vi "Camera Main.vi"() -> ()   [LabVIEW 2013]
uses:
  Controls/Controls Tab.ctl
  <vilib>/Utility/miscctls.llb/LVRectTypeDef.ctl
  GUI_Template/GUI_master/tcp_new_data_event.ctl
  GUI_Template/GUI_master/tcp new data cluster.ctl
  color tables/image color table presets.ctl
  Controls/IMAQ control.ctl
  <vilib>/vision/Image Controls.llb/IMAQ Image.ctl
  Controls/IMG Features.ctl
  Controls/TCP Cluster.ctl
  <vilib>/vision/NI_Vision_Development_Module.lvlib
panel:
  out "fast ID (h)":refnum<k16>
  out "slow ID (h)":refnum<k16>
  in  "Color table":T1=enum."BWR enhance low"
  in  "Maximize!!":bool
  out "error message":string
  out "Device Name (h)":string="FakeCam1"
  in  "Hide controls":bool
  out "image::1":T2(plugin-control) caption="HPD_CCD"
  in  "File Path":path
  out "error IO 2":errorcluster
  out "tcp data event":T3
  in  "Tab Control":T4
  in  "size 2":cluster{"xhair size":dbl, "xhair size 2":dbl}={"xhair size"=20.0, "xhair size 2"=20.0} {"xhair size 2" min=0.0 max=0.0; "xhair size" min=0.0 max=0.0}
  in  "Target.X":dbl caption="TargetX"
  in  "Target.Y":dbl caption="TargetY"
  in  "draw Xhair":bool
  in  "Scale":bool
  in  "Autoscale":bool
  in  "String":string="M1Cam"
  in  "GUIdevice 1":string="HPD_CCD"
  in  "stop":bool
  in  "scale factor":dbl=2.0 caption="Scale factor"
  in  "Trigger":bool
  in  "Save":bool
  in  "Gain":dbl
  in  "exposure":dbl=0.52 caption="Exposure"
  in  "Triggerdelay":dbl
  in  "Fit Control":bool
  in  "Shotnumber":i32=354
  out "Max Counts":dbl(slide) scale=0.0..256.0
  in  "Size & Tolerance":T5={"X Size"=5, "Y Size"=5, "% Tolerance"=100}
  in  "LowPass":bool
  in  "Sat Level":sgl=255.0
  out "Mean Value":sgl format="%.2f"
  in  "Beep If Sat.":bool
  in  "MaxGUIPixel":dbl
  in  "ROI.Width":dbl
  in  "ROI.Height":dbl
  in  "ROI.OffsetX":dbl
  in  "ROI.OffsetY":dbl
  out "Centroid":cluster{"X Centroid":sgl, "Y Centroid":sgl} {"Y Centroid" format="%.2f"; "X Centroid" format="%.2f"}
  out "Y Resolution":i32
  out "X Resolution":i32
  out "GUIBinning":dbl
  out "Mean Value Graph":sgl(graph)
  out "histogram":T6(graph)
  out "lineout":cluster{"x0":sgl, "dx":sgl, "Pixels Line":sgl[]}(graph)
  out "MaxCounts":dbl
  in  "SpatialCalibration":dbl
  in  "FWHMx":dbl
  in  "FWHMy":dbl
  out "FWHMx (um)":dbl
  out "FWHMy (um)":dbl
  in  "Analysis":bool
  out "MeanCounts":dbl
  in  "localsavingpath":path
  in  "time to wait (TCP)":i32=10
  in  "send":bool
  in  "reset":bool
  in  "Timeout ms (slow resp)":i32=500
  out "port or service name":u16=65400
  out "local Port":u16=65401
  out "connections (hidden)":variant[](array[variant])=[variant(refnum<k16> refnum), variant(refnum<k16> refnum)]
  out "Data connection ok":bool
  out "Image connection":bool
  out "error (h)":bool
  out "centroidy 2":dbl
  out "centroidy":dbl
  out "Remote Host":string="192.168.10.157"
  out "Top":i16
  out "Left":i16
  out "Content Area Rect":T7
  out "Image (IMAQ)":T2(plugin-control)
  # "Unused controls Do not Delete"
  # "Crosshair"
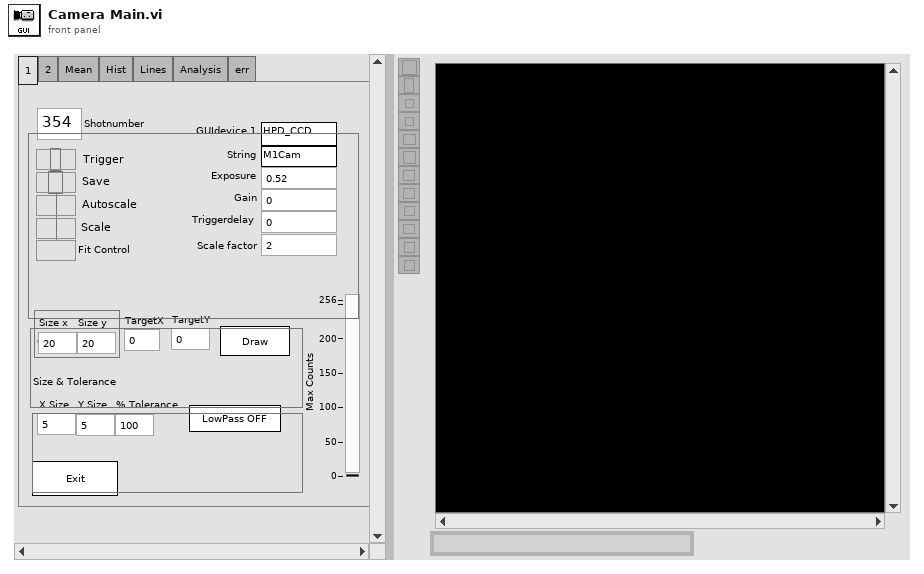
[diagram p1: front panel]
types:
  T1 = typedef "image color table presets.ctl" = enum16{"enhance low", "blue yellow red", "BYR enhance low", "white blue yellow", "BWR enhance low", "make a new one"}
  T2 = typedef "IMAQ Image.ctl" = refnum<image>
  T3 = typedef "tcp_new_data_event.ctl" = refnum<user-event>
  T4 = typedef "Controls Tab.ctl" = enum32{"1", "2", "Mean", "Hist", "Lines", "Analysis", "err"}
  T5 = cluster{"X Size":i32, "Y Size":i32, "% Tolerance":i32}
  T6 = cluster{"Starting Value":sgl, "Incremental Value":sgl, "Histogram":u32[]}
  T7 = typedef "LVRectTypeDef.ctl" = cluster{"Left":i16, "Top":i16, "Right":i16, "Bottom":i16}
  T8 = typedef "EventTypDef.ctl" = refnum<user-event>
  T9 = enum32{"Invalid", "Standard", "Closed", "Hidden", "Minimized", "Maximized"}
  T10 = enum32{"invalid app kind", "Development System", "Run Time System", "Student Edition", "Embedded LabVIEW", "Evaluation", "Custom"}
  T11 = cluster{"Left":i32, "Top":i32, "Right":i32, "Bottom":i32}
  T12 = typedef "IMAQ control.ctl" = cluster{"Image Out":T2, "valid image":bool, "X resolution":i32, "Y resolution":i32, "Image Area":cluster{"Width":u32, "Height":u32}, "zoom to fit":bool, "Image Center":cluster{"X":u32, "Y":u32}, "Max count":dbl}
  T13 = typedef "IMG Features.ctl" = cluster{"Color table":T1, "Button Label":string}
  T14 = typedef "TCP Cluster.ctl" = cluster{"Port":u16, "Remote Host":string, "All Devices":string[], "New Device":bool}
  T15 = cluster{"Core":cluster{"Current VI Reference":refnum<vi>, "Close Panel on Exit?":bool}, "tcp connections":refnum<k5>[], "subscribe messages":string[], "Image Data":T12, "images":T2[], "IMG Features":T13, "TCP Cluster":T14}
  T16 = typedef "Image Type" = u32
  T17 = cluster{"Current VI Reference":refnum<vi>, "Close Panel on Exit?":bool}
  T18 = cluster{"Global Rectangle":i32[], "Contours":cluster{"Contour Type":u32, "ROI Type":u32, "Points":i32[]}[]}
  T19 = typedef "IMAQ Line" = cluster{"Start X":i32, "Start Y":i32, "End X":i32, "End Y":i32}
  T20 = typedef "tcp new data cluster.ctl" = cluster{"EventEnum":enum16{"new data", "connection status update"}, "Device name":string}
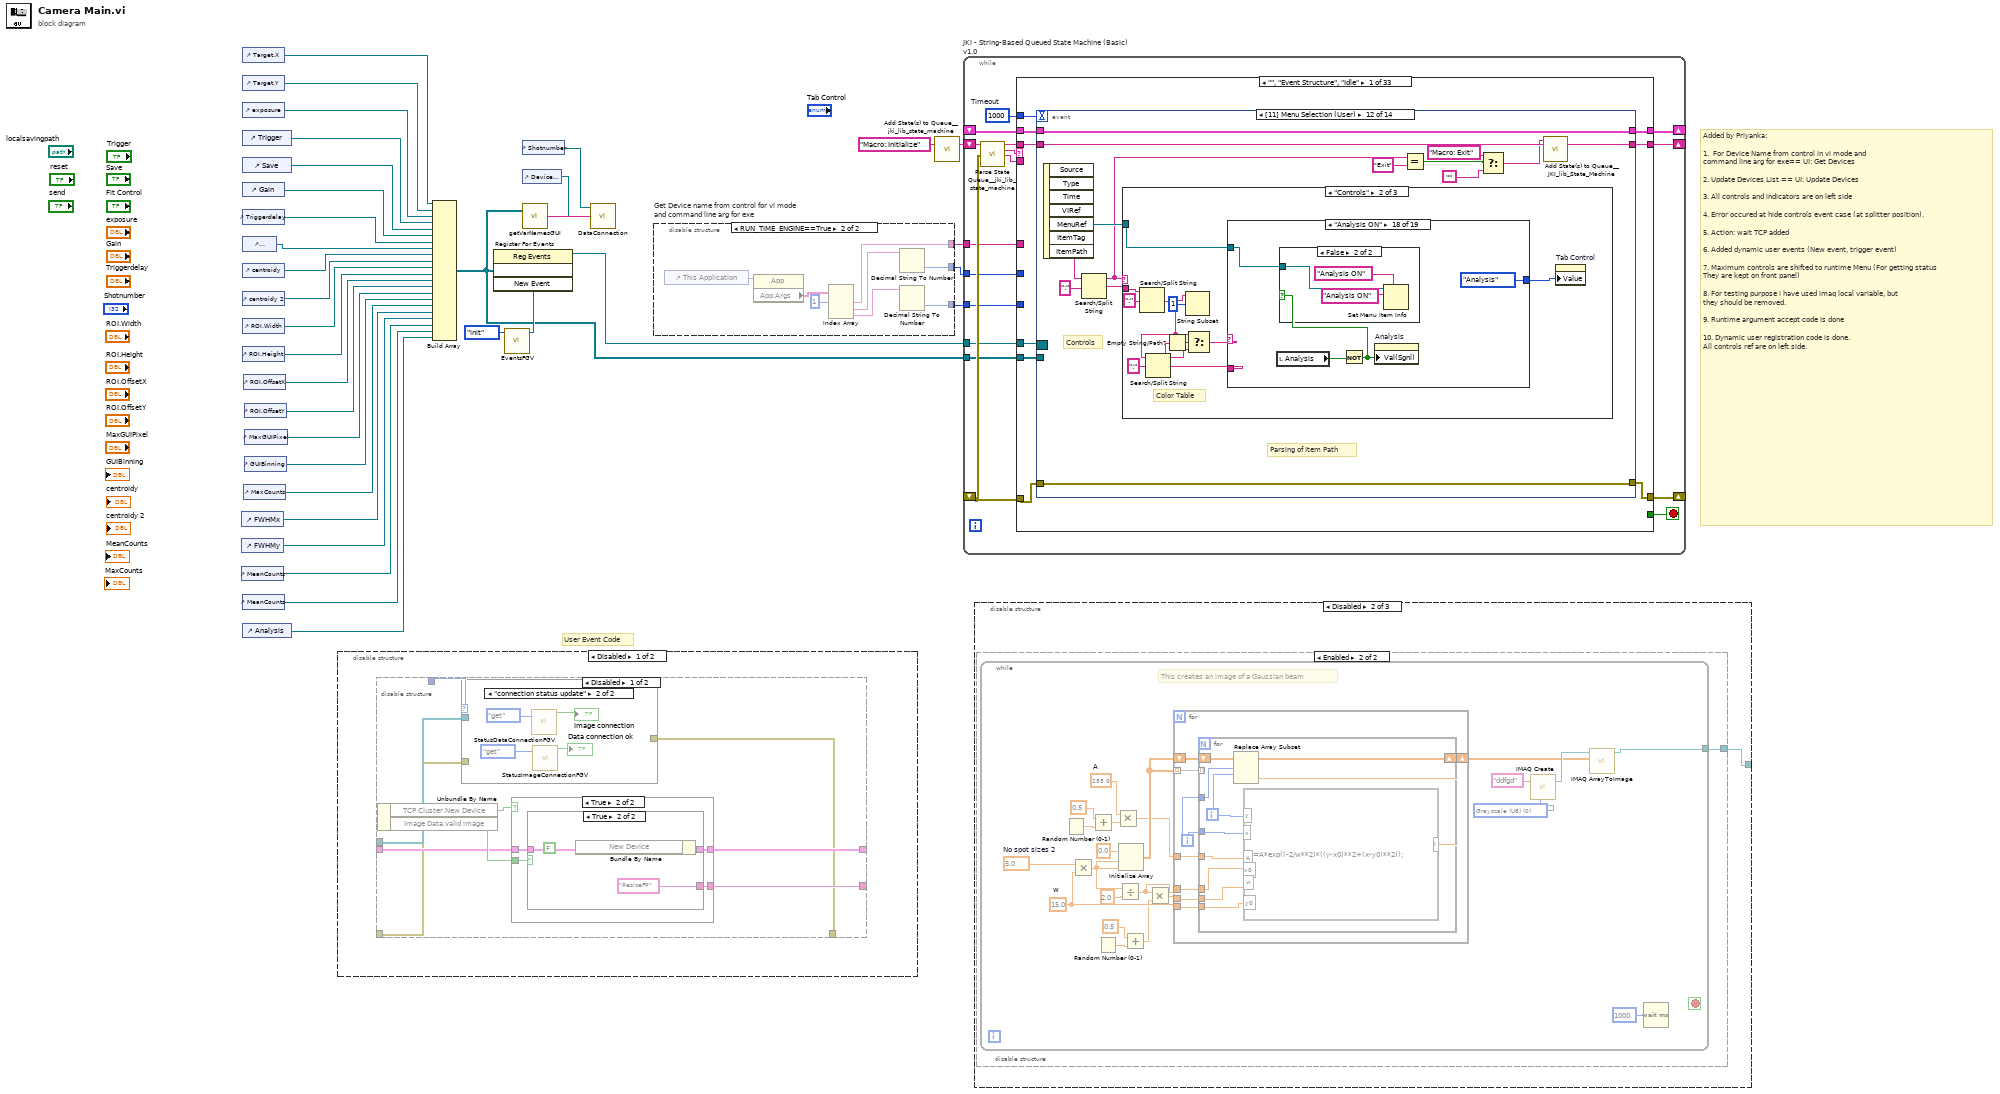
[diagram p0: block diagram]
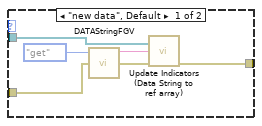
[diagram p4: hidden frame]
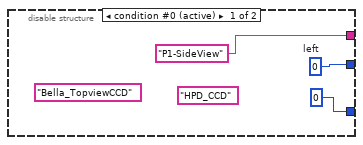
[diagram p7: hidden frame]
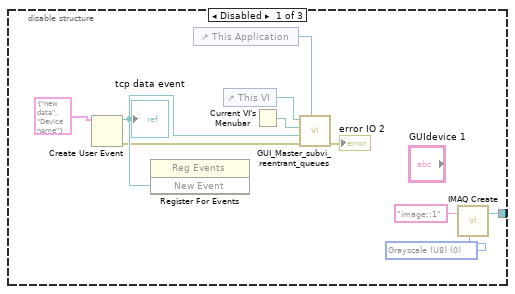
[diagram p8: hidden frame]
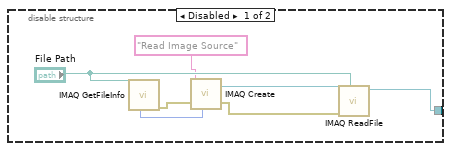
[diagram p9: hidden frame]
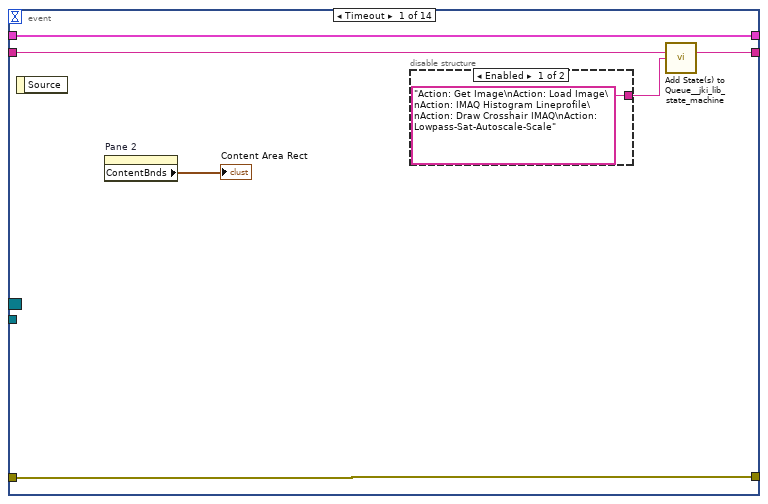
[diagram p11: hidden frame]
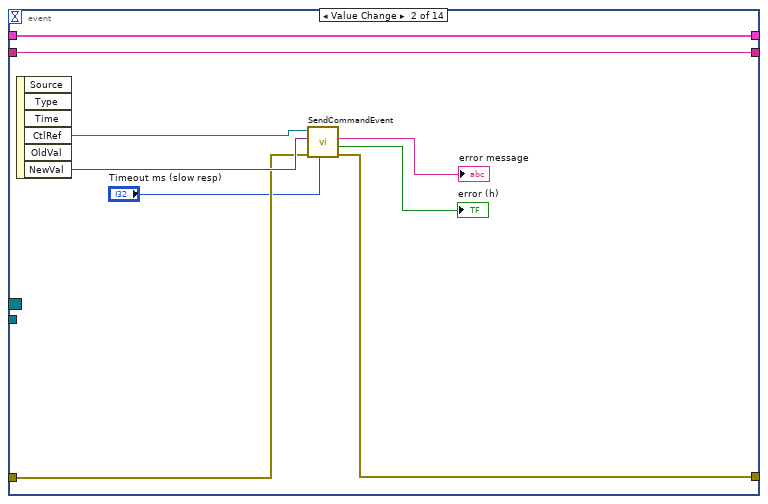
[diagram p13: hidden frame]
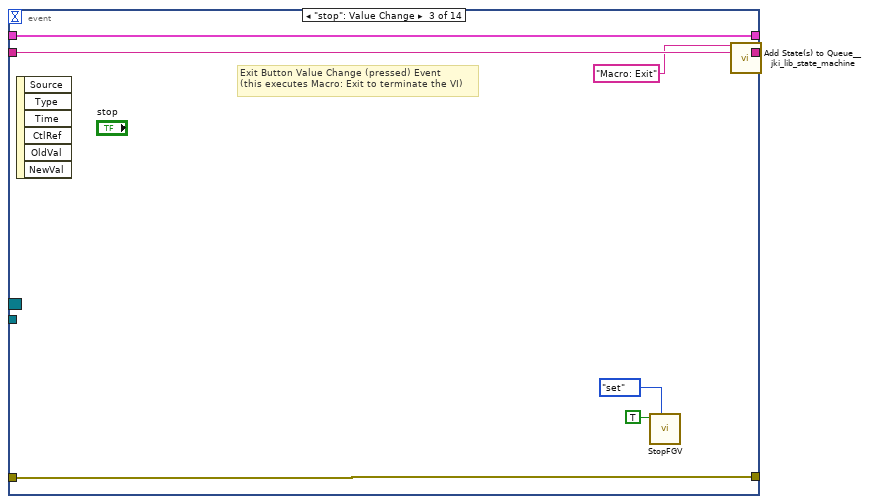
[diagram p14: hidden frame]
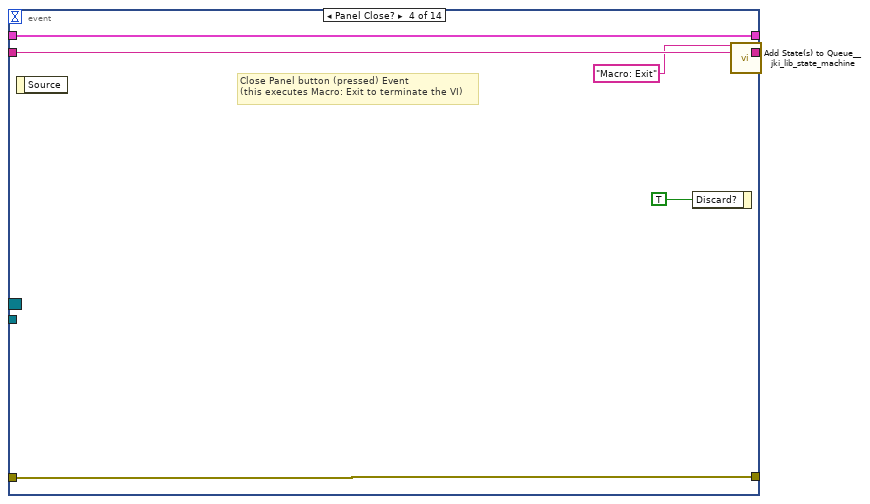
[diagram p15: hidden frame]
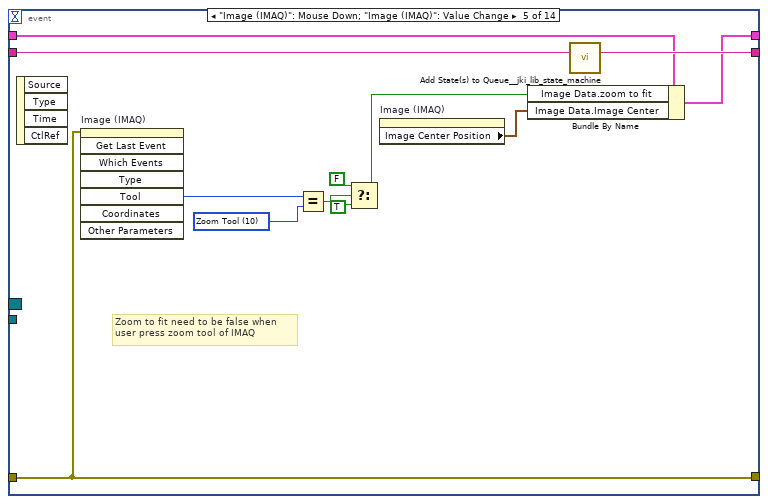
[diagram p16: hidden frame]
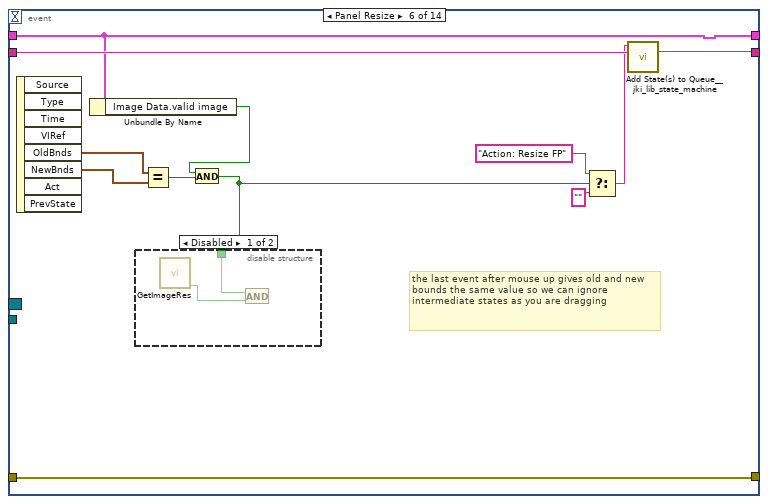
[diagram p17: hidden frame]
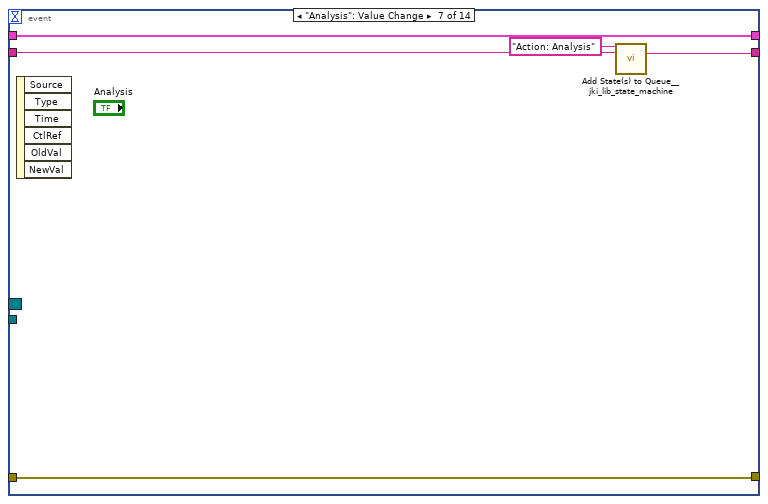
[diagram p19: hidden frame]
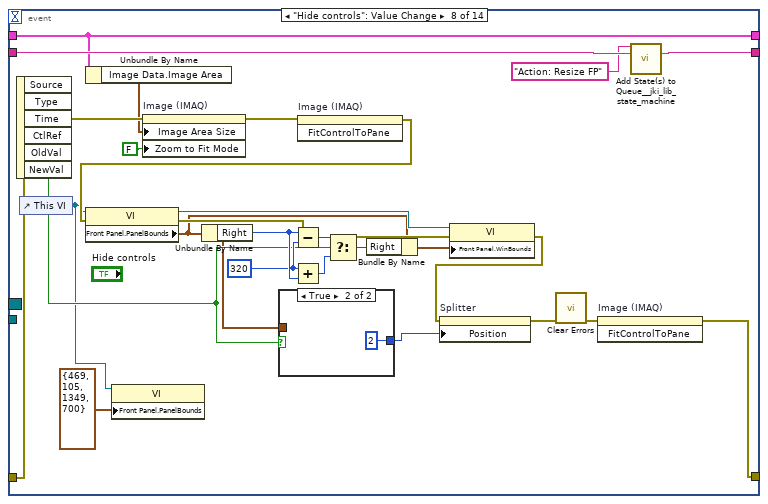
[diagram p20: hidden frame]
diagram:
  # "User Event Code"
  # "Added by Priyanka:\n\n1.  For Device Name from control in vi mode and \ncommand line arg for exe== UI: Get Devices\n\n2. Update Devices List == UI: Update Devices\n\n3. All controls and indicators are on left side\n\n4. Error occured at hide controls event case (at splitter position).\n\n5. Action: wait TCP added\n\n6. Added dynamic user events (New event, trigger event)\n\n7. Maximum controls are shifted to runtime Menu (For getting status\nThey are kept on front panel)\n\n8. For testing purpose i have used imaq local variable, but \nthey should be removed.\n\n9. Runtime argument accept code is done\n\n10. Dynamic user registration code is done. \nAll controls ref are on left side."
  n1 = control-ref of="FWHMx"() -> (w9:refnum<vi>)
  n2 = control-ref of="FWHMy"() -> (w8:refnum<vi>)
  n3 = control-ref of="MeanCounts"() -> (w7:refnum<vi>)
  n4 = control-ref of="Target.X"() -> (w26:refnum<vi>)
  n5 = control-ref of="Target.Y"() -> (w25:refnum<vi>)
  n6 = control-ref of="exposure"() -> (w24:refnum<vi>)
  n7 = control-ref of="Trigger"() -> (w23:refnum<vi>)
  n8 = control-ref of="Save"() -> (w22:refnum<vi>)
  n9 = control-ref of="Gain"() -> (w21:refnum<vi>)
  n10 = control-ref of="Triggerdelay"() -> (w20:refnum<vi>)
  n11 = control-ref of="localsavingpath"() -> (w15:refnum<vi>)
  n12 = control-ref of="centroidy"() -> (w19:refnum<vi>)
  n13 = control-ref of="centroidy 2"() -> (w18:refnum<vi>)
  n14 = control-ref of="ROI.Width"() -> (w17:refnum<vi>)
  n15 = control-ref of="ROI.Height"() -> (w16:refnum<vi>)
  n16 = control-ref of="MeanCounts"() -> (w6:refnum<vi>)
  n17 = control-ref of="Analysis"() -> (w5:refnum<vi>)
  n18 = control-ref of="ROI.OffsetX"() -> (w14:refnum<vi>)
  n19 = control-ref of="MaxCounts"() -> (w10:refnum<vi>)
  n20 = control-ref of="ROI.OffsetY"() -> (w13:refnum<vi>)
  n21 = control-ref of="GUIBinning"() -> (w11:refnum<vi>)
  n22 = control-ref of="MaxGUIPixel"() -> (w12:refnum<vi>)
  n23 = disable-structure shown="Disabled" {
    frame Disabled {
      n24 = disable-structure shown="Disabled" {
        disable-tunnel: _ -> [w43 _]
        disable-tunnel: _ -> [w42 _]
        disable-tunnel: [w39 _] -> _
        disable-tunnel: _ -> [w38 _]
        disable-tunnel: [w37 _] -> _
        disable-tunnel: [w36 _] -> _
        disable-tunnel: _ -> [w35 _]
        frame Disabled {
          n25 = Unbundle By Name() -> ("TCP Cluster.New Device"=w40:bool, "Image Data.valid image"=w41:bool)  [unwired: 1 in]
          n26 = case shown="\"connection status update\"" w42 {
            tunnel: w43 -> [w57 _]
            tunnel: [w55 _] -> w36
            tunnel: w35 -> [w54 _]
            frame "new data", Default {
              n27 = call "DATAStringFGV.vi"("Command"=enum16{"get", "set", "init"}."get") -> ("Data String out"=w56:string)  [unwired: 9 in, 1 out]
              n28 = call "Update Indicators (Data String to ref array).vi"("Array"=w57, "Data String"=w56, "error in (no error)"=w54) -> ("error out"=w55:errorcluster)  [unwired: 11 in, 1 out]
            }
            frame "connection status update" {
              n29 = call "StatusDataConnectionFGV.vi"("Command"=enum16{"get", "set", "init"}."get") -> ("Data Connection out"=→"Image connection":bool)  [unwired: 10 in]
              n30 = call "StatusImageConnectionFGV.vi"("Command"=enum16{"get", "set", "init"}."get") -> ("Image Connection out"=→"Data connection ok":bool)  [unwired: 10 in]
            }
          }
          n31 = case shown="True" w40 {
            tunnel: [_ w48] -> w39
            tunnel: w41 -> [_ w47]
            tunnel: w38 -> [w44 w46]
            tunnel: [w44 w45] -> w37
            frame False {
            }
            frame True {
              n32 = case shown="True" w47 {
                tunnel: [_ "ResizeFP" ("State(s) in (\"\")")] -> w48
                tunnel: w46 -> [w49 w52]
                tunnel: [w49 w51] -> w45
                frame False {
                }
                frame True {
                  n33 = Bundle By Name(cluster=w52, "New Device"=FALSE ("new device")) -> (w51:cluster{})
                }
              }
            }
          }
        }
        frame Enabled {
        }
      }
    }
    frame Enabled {
    }
  }
  n34 = Build Array(w26, w25, w24, w23, w22, w21, w20, w15, w19, w18, w17, w16, w14, w13, w12, w11, w10, w9, w8, w7, w6, w5) -> (w3:refnum<vi>[])
  n35 = call "EventsFGV.vi"("Command"=enum16{"get", "init"}."init") -> ("New Event"=w27:T8)  [unwired: 9 in, 1 out]
  n36 = register-events(w3, w27) -> (reference out=w4:refnum<event-registration>)  [unwired: 2 in, 1 out]
  n37 = control-ref of="Shotnumber"() -> (w2:refnum<vi>)
  n38 = control-ref of="Device Name (h)"() -> (w1:refnum<vi>)
  n39 = call "getVarNamesGUI.vi"("Array"=w3) -> ("String"=w29:string)  [unwired: 1 in]
  n40 = call "DataConnection.vi"("Subscriber list"=w29, "Device Name (h)"=w1, "shotnumber"=w2) -> ()
  n41 = disable-structure "Get Device name from control for vi mode\nand command line arg for exe" shown="RUN_TIME_ENGINE==True" {
    disable-tunnel: ["P1-SideView" ("Device Name for vi mode") w70] -> w32
    disable-tunnel: [w64 w67] -> w30
    disable-tunnel: [i16 0 ("left") w66] -> w31
    frame condition #0 (active) {
      (unwired) "Bella_TopviewCCD" ("Device Name for vi mode")
      (unwired) "HPD_CCD" ("Device Name for vi mode")
      w64 = i16 0  # left
    }
    frame condition #1 {
      n42 = control-ref of="This Application"() -> (w73:refnum<vi>)
      n43 = property class="App"(reference=w73) -> ("App.Args"=w72:string[])  [unwired: 1 in, 2 out]
      n44 = Index Array(array=w72, index #1=1 ("index")) -> (element #1=w70:string, element #2=w69:string, element #3=w68:string)  [unwired: 2 in]
      n45 = Decimal String To Number(string=w69) -> (number=w67:i32)  [unwired: 2 in, 1 out]
      n46 = Decimal String To Number(string=w68) -> (number=w66:i32)  [unwired: 2 in, 1 out]
    }
  }
  n47 = call <vilib>:"Add State(s) to Queue__jki_lib_state_machine.vi"("State(s) in (\"\")"="Macro: Initialize") -> ("States Out"=w34:string)  [unwired: 14 in]
  n48 = while "JKI - String-Based Queued State Machine (Basic) v1.0" {
    shift-right: [w82] -> _
    shift-left: _ -> [w81]
    shift-right: [w85] -> _
    shift-left: _ -> [w79]
    shift-right: [w84] -> _
    shift-left: w34 -> [w86]
    tunnel: w32 -> [w78]
    tunnel: w31 -> [w77]
    tunnel: w30 -> [w76]
    tunnel: w4 -> [w75]
    tunnel: w3 -> [w74]
    stop <- w83 stop-if-true
    w80 = 1000  # Timeout
    n49 = call <vilib>:"Parse State Queue__jki_lib_state_machine.vi"("State Queue"=w86, "Error In (no error)"=w79) -> ("Remaining States"=w88:string, "Current State"=w89:string, "Arguments"=w87:string)  [unwired: 11 in]
    n50 = case shown="\"\", \"Event Structure\", \"Idle\"" w89 {
      selector: w89 -> [_ _ w380 _ _ _ _ _ _ _ _ _ _ _ _ _ _ _ _ _ _ _ _ _ _ _ _ _ _ _ _ _ _]
      tunnel: w88 -> [w98 w379 w384 w402 w408 w413 w417 w432 w447 w451 w462 w475 w488 w506 w512 w523 w549 w554 w559 w569 w573 w583 w608 w630 w640 w664 w698 w721 w745 w763 w779 w810 w853]
      tunnel: w87 -> [_ _ _ _ _ _ _ _ _ _ _ _ _ _ w507 w517 _ _ _ _ _ _ _ _ _ _ _ _ _ _ _ _ _]
      tunnel: w81 -> [w96 w376 w382 w393 w405 w411 w414 _ w444 w448 w455 w466 w478 w500 w510 w519 w546 w551 w556 w566 w570 w578 w586 w631 w633 w671 w718 w728 w748 w760 w783 w805 w854]
      tunnel: [w95 w377 w386 w399 errorcluster {"status"=FALSE, "code"=0, "source"=""} ("error out") w410 w415 w429 w433 w449 w460 w474 w487 w505 w508 w520 w547 w552 w557 w567 w571 w581 w607 w629 w635 w665 w717 w729 w750 w755 w785 w809 w852] -> w85
      tunnel: w79 -> [w94 w377 w385 w399 w404 w410 w415 w429 w436 w449 w460 w474 w487 w505 w509 w521 w547 w552 w557 w567 w571 w581 w607 w629 w636 w666 w716 w723 w750 w756 w785 w809 w852]
      tunnel: [w97 w378 w383 w401 w407 w412 w416 w431 w446 w450 w461 w475 w488 w506 w511 w522 w548 w553 w558 w568 w572 w582 w608 w630 w639 w663 w698 w721 w745 w763 w779 w810 w853] -> w84
      tunnel: [_ _ _ _ _ TRUE _ _ _ _ _ _ _ _ _ _ _ _ _ _ _ _ _ _ _ _ _ _ _ _ _ _ _] -> w83
      tunnel: [w93 w376 w382 w400 w405 w411 w414 w430 w444 w448 w454 w465 w477 w500 w510 w519 w546 w551 w556 w566 w570 w577 w585 w631 w638 w670 w718 w727 w748 w759 w782 w804 w854] -> w82
      tunnel: w80 -> [w92 _ _ _ _ _ _ _ _ _ _ _ _ _ _ _ _ _ _ _ _ _ _ _ _ _ _ _ _ _ _ _ _]
      tunnel: w78 -> [_ _ _ _ _ _ _ _ _ _ _ w469 _ _ _ _ _ _ _ _ _ _ _ _ _ _ _ _ _ _ _ _ _]
      tunnel: w77 -> [_ _ _ _ _ _ _ _ _ _ _ w468 _ _ _ _ _ _ _ _ _ _ _ _ _ _ _ _ _ _ _ _ _]
      tunnel: w76 -> [_ _ _ _ _ _ _ _ _ _ _ w467 _ _ _ _ _ _ _ _ _ _ _ _ _ _ _ _ _ _ _ _ _]
      tunnel: w75 -> [w91 _ _ _ _ _ _ _ _ _ _ _ _ _ _ _ _ _ _ _ _ _ _ _ _ _ _ _ _ _ _ _ _]
      tunnel: w74 -> [w90 _ _ _ _ _ _ _ _ _ _ _ _ _ _ _ _ _ _ _ _ _ _ _ _ _ _ _ _ _ _ _ _]
      frame "", "Event Structure", "Idle" {
        n51 = event shown="[11] Menu Selection (User)" {
          selector: w91 -> [_ _ _ _ _ _ _ _ _ _ _ _ _ _]
          dyn-events: _ -> [_ _ _ _ _ _ _ _ _ _ _ _ _ _]
          timeout: w92 -> [_ _ _ _ _ _ _ _ _ _ _ _ _ _]
          tunnel: w98 -> [w104 w113 w121 w127 w138 w150 w156 w170 w189 w197 w206 w216 w356 w374]
          tunnel: [w103 w113 w120 w126 w139 w151 w157 w169 w190 w196 w205 w215 w355 w374] -> w97
          tunnel: w96 -> [w99 w114 w118 w124 w137 w142 w159 w160 w194 w199 w202 w220 w362 w375]
          tunnel: [w102 w107 w119 w125 w130 w149 w158 w174 w191 w198 w204 w221 w357 w372] -> w95
          tunnel: w94 -> [w102 w108 w119 w125 w130 w149 w158 w172 w191 w198 w204 w221 w358 w373]
          tunnel: [w99 w114 w118 w124 w128 w142 w159 w160 w193 w199 w201 w220 w362 w375] -> w93
          tunnel: w90 -> [_ _ _ _ _ _ _ _ _ _ _ _ _ _]
          event Timeout {
            n52 = event-data() -> ()  [unwired: 1 in, 1 out]
            n53 = property on="Pane 2" class="Pane"() -> ("ContentBnds"=→"Content Area Rect":T7)  [unwired: 2 in, 2 out]
            n54 = disable-structure shown="Enabled" {
              disable-tunnel: ["Action: Get Image\nAction: Load Image\nAction: IMAQ Histogram Lineprofile\nAction: Draw Crosshair IMAQ\nAction: Lowpass-Sat-Autoscale-Scale" ("State(s) in Front (\"\")") _] -> w100
              frame Enabled {
              }
              frame Disabled {
              }
            }
            n55 = call <vilib>:"Add State(s) to Queue__jki_lib_state_machine.vi"("State(s) in (\"\")"=w104, "State(s) at Back (\"\")"=w100) -> ("States Out"=w103:string)  [unwired: 13 in]
          }
          event Value Change {
            n56 = event-data() -> ("CtlRef"=w112:refnum<vi>, "NewVal"=w111:variant)  [unwired: 1 in, 4 out]
            n57 = call "SendCommandEvent.vi"("timeout ms (slow resp)"="Timeout ms (slow resp)", "error out 2"=w108, "NewVal"=w111, "CtlRef"=w112) -> ("error out"=w107:errorcluster, "error (h)"=→"error (h)":bool, "error message"=→"error message":string)  [unwired: 4 in, 1 out]
          }
          event "stop": Value Change {
            # "Exit Button Value Change (pressed) Event\n(this executes Macro: Exit to terminate the VI)"
            n58 = event-data() -> ()  [unwired: 1 in, 6 out]
            n59 = call "StopFGV.vi"("Command"=enum16{"set", "get", "init"}."set", "Stop"=TRUE) -> ()  [unwired: 9 in, 1 out]
            n60 = call <vilib>:"Add State(s) to Queue__jki_lib_state_machine.vi"("State(s) in Front (\"\")"="Macro: Exit", "State(s) in (\"\")"=w121) -> ("States Out"=w120:string)  [unwired: 13 in]
          }
          event Panel Close? {
            # "Close Panel button (pressed) Event\n(this executes Macro: Exit to terminate the VI)"
            n61 = event-data() -> ()  [unwired: 1 in, 1 out]
            n62 = event-data("Discard?"=TRUE) -> ()  [unwired: 1 in, 1 out]
            n63 = call <vilib>:"Add State(s) to Queue__jki_lib_state_machine.vi"("State(s) in Front (\"\")"="Macro: Exit", "State(s) in (\"\")"=w127) -> ("States Out"=w126:string)  [unwired: 13 in]
          }
          event "Image (IMAQ)": Mouse Down; "Image (IMAQ)": Value Change {
            w136 = 10 items=["None", "Selection Tool", "Point Tool", "Line Tool", "Rectangle Tool", "Oval Tool", "Polygon Tool", "ClosedFreehandTool", "Annulus Tool", "Rotated Rectangle Tool", "Zoom Tool", "Pan Tool", "Polyline Tool", "Freehand Tool"] ("Tool")
            # "Zoom to fit need to be false when \nuser press zoom tool of IMAQ"
            n64 = event-data() -> ()  [unwired: 1 in, 4 out]
            n65 = invoke on="Image (IMAQ)" class="ImageControl" method="Get Last Event"(error in=w130) -> ("Tool"=w135:i32)  [unwired: 7 in, 7 out]
            n66 = Equal?(x=w135, y=w136) -> (x = y?=w132:bool)
            n67 = Select(t=FALSE, s=w132, f=TRUE) -> (s? t:f=w131:bool)
            n68 = property on="Image (IMAQ)" class="ImageControl"() -> ("Image Center Position"=w129:cluster{"X":u32, "Y":u32})  [unwired: 2 in, 2 out]
            n69 = Bundle By Name(cluster=w137, "Image Data.zoom to fit"=w131, "Image Data.Image Center"=w129) -> (w128:T15)
            n70 = call <vilib>:"Add State(s) to Queue__jki_lib_state_machine.vi"("State(s) in (\"\")"=w138) -> ("States Out"=w139:string)  [unwired: 14 in]
          }
          event Panel Resize {
            # "the last event after mouse up gives old and new bounds the same value so we can ignore intermediate states as you are dragging"
            n71 = event-data() -> ("OldBnds"=w148:T7, "NewBnds"=w147:T7)  [unwired: 1 in, 6 out]
            n72 = Unbundle By Name(w142) -> ("Image Data.valid image"=w141:bool)
            n73 = Equal?(x=w148, y=w147) -> (x = y?=w143:bool)
            n74 = And(x=w141, y=w143) -> (x .and. y?=w140:bool)
            n75 = disable-structure shown="Disabled" {
              disable-tunnel: w140 -> [w153 _]
              frame Disabled {
                n76 = call "GetImageRes.vi"() -> ("valid Image"=w152:bool, "Image Area:Size:All Elements"=w154:cluster{"Width":u32, "Height":u32})  [unwired: 7 in, 3 out]
                n77 = And(x=w153, y=w152) -> ()  [unwired: 1 out]
              }
              frame Enabled {
              }
            }
            n78 = Select(t="Action: Resize FP" ("State(s) in Front (\"\")"), s=w140, f="" ("t")) -> (s? t:f=w144:string)
            n79 = call <vilib>:"Add State(s) to Queue__jki_lib_state_machine.vi"("State(s) in Front (\"\")"=w144, "State(s) in (\"\")"=w150) -> ("States Out"=w151:string)  [unwired: 13 in]
          }
          event "Analysis": Value Change {
            n80 = event-data() -> ()  [unwired: 1 in, 6 out]
            n81 = call <vilib>:"Add State(s) to Queue__jki_lib_state_machine.vi"("State(s) in Front (\"\")"="Action: Analysis" ("State(s) in Front (\"\")"), "State(s) in (\"\")"=w156) -> ("States Out"=w157:string)  [unwired: 13 in]
          }
          event "Hide controls": Value Change {
            w181 = 320 ("Position:Left")
            n82 = event-data() -> ("NewVal"=w180:bool)  [unwired: 1 in, 5 out]
            n83 = control-ref of="This VI"() -> (w164:refnum<vi>)
            n84 = Unbundle By Name(w160) -> ("Image Data.Image Area"=w171:cluster{"Width":u32, "Height":u32})
            n85 = property class="VI"(reference=w164, "Front Panel.PanelBounds"=T7 {"Left"=469, "Top"=105, "Right"=1349, "Bottom"=700} ("Front Panel Window:Panel Bounds")) -> ()  [unwired: 1 in, 2 out]
            n86 = property on="Image (IMAQ)" class="ImageControl"(error in=w172, "Image Area Size"=w171, "Zoom to Fit Mode"=FALSE) -> (error out=w165:errorcluster)  [unwired: 1 in, 1 out]
            n87 = invoke on="Image (IMAQ)" class="ImageControl" method="FitControlToPane"(error in=w165) -> (error out=w173:errorcluster)  [unwired: 2 in, 2 out]
            n88 = property class="VI"(reference=w164, error in=w173) -> (reference out=w178:refnum<vi>, error out=w177:errorcluster, "Front Panel.PanelBounds"=w162:T7)
            n89 = Unbundle By Name(w162) -> ("Right"=w182:i16)
            n90 = case shown="True" w180 {
              tunnel: [372 ("Position:Left") 2 ("Position:Left")] -> w176
              tunnel: w162 -> [_ _]
              frame False {
              }
              frame True {
              }
            }
            n91 = Subtract(x=w182, y=w181) -> (x-y=w183:i32)
            n92 = Add(x=w181, y=w182) -> (x+y=w184:i32)
            n93 = Select(t=w183, s=w180, f=w184) -> (s? t:f=w185:i32)
            n94 = Bundle By Name(cluster=w162, "Right"=w185) -> (w179:T7)
            n95 = property class="VI"(reference=w178, error in=w177, "Front Panel.WinBounds"=w179) -> (error out=w163:errorcluster)  [unwired: 1 out]
            n96 = property on="Splitter" class="Splitter"(error in=w163, "Position"=w176) -> (error out=w175:errorcluster)  [unwired: 1 in, 1 out]
            n97 = call <vilib>:"Clear Errors.vi"("error in (no error)"=w175) -> ("error out"=w167:errorcluster)  [unwired: 6 in]
            n98 = invoke on="Image (IMAQ)" class="ImageControl" method="FitControlToPane"(error in=w167) -> (error out=w174:errorcluster)  [unwired: 2 in, 2 out]
            n99 = call <vilib>:"Add State(s) to Queue__jki_lib_state_machine.vi"("State(s) in Front (\"\")"="Action: Resize FP", "State(s) in (\"\")"=w170) -> ("States Out"=w169:string)  [unwired: 13 in]
          }
          event Value Change {
            n100 = event-data() -> ()  [unwired: 1 in, 6 out]
            n101 = Bundle By Name(cluster=w194, "IMG Features.Color table"="Color table") -> (w193:T15)
            n102 = call <vilib>:"Add State(s) to Queue__jki_lib_state_machine.vi"("State(s) in Front (\"\")"="Action: Color Table", "State(s) in (\"\")"=w189) -> ("States Out"=w190:string)  [unwired: 13 in]
          }
          event "draw Xhair": Value Change {
            n103 = event-data() -> ()  [unwired: 1 in, 6 out]
            n104 = call <vilib>:"Add State(s) to Queue__jki_lib_state_machine.vi"("State(s) in Front (\"\")"="Action: Draw Crosshair IMAQ", "State(s) in (\"\")"=w197) -> ("States Out"=w196:string)  [unwired: 13 in]
          }
          event "Beep If Sat.", "LowPass", "Autoscale", "Scale": Value Change {
            n105 = event-data() -> ("CtlRef"=w203:refnum<vi>)  [unwired: 1 in, 5 out]
            n106 = property class="Bool (strict)"(reference=w203) -> ("Label.Text"=w200:string)  [unwired: 1 in, 2 out]
            n107 = Bundle By Name(cluster=w202, "IMG Features.Button Label"=w200) -> (w201:T15)
            n108 = call <vilib>:"Add State(s) to Queue__jki_lib_state_machine.vi"("State(s) in Front (\"\")"="Action: IMAQ Histogram Lineprofile\nAction: Lowpass-Sat-Autoscale-Scale", "State(s) in (\"\")"=w206) -> ("States Out"=w205:string)  [unwired: 13 in]
          }
          event Menu Selection (User) {
            # "Parsing of Item Path"
            # "Controls"
            n109 = event-data() -> ("MenuRef"=w217:refnum<k9>, "ItemPath"=w219:string)  [unwired: 1 in, 5 out]
            n110 = Search/Split String(string=w219, search string/char (-)=":") -> (substring before match=w208:string, match + rest of string=w214:string)  [unwired: 1 in, 1 out]
            n111 = case shown="\"Controls\"" w208 {
              tunnel: w214 -> [_ w231 _]
              tunnel: w217 -> [_ w232 _]
              frame "False", Default {
              }
              frame "Controls" {
                # "Color Table"
                n112 = Search/Split String(string=w231, search string/char (-)=":") -> (match + rest of string=w230:string)  [unwired: 1 in, 2 out]
                n113 = String Subset(string=w230, offset (0)=1) -> (substring=w225:string)  [unwired: 1 in]
                n114 = Search/Split String(string=w225, search string/char (-)=":") -> (substring before match=w226:string, match + rest of string=w223:string)  [unwired: 1 in, 1 out]
                n115 = Empty String/Path?(string/path=w226) -> (empty?=w227:bool)
                n116 = Select(t=w225, s=w227, f=w226) -> (s? t:f=w224:string)
                n117 = case shown="\"Analysis ON\"" w224 {
                  selector: w224 -> [_ _ _ _ _ _ _ _ w243 _ _ _ _ _ _ _ _ _ _]
                  tunnel: [_ Controls_Tab."1" ("Tab Control") Controls_Tab."2" ("Tab Control") Controls_Tab."Mean" ("Tab Control") Controls_Tab."Hist" ("Tab Control") Controls_Tab."Lines" ("Tab Control") Controls_Tab."Analysis" ("Tab Control") Controls_Tab."err" ("Tab Control") Controls_Tab."1" ("Tab Control") Controls_Tab."1" ("Tab Control") Controls_Tab."1" ("Tab Control") Controls_Tab."1" ("Tab Control") _ Controls_Tab."1" ("Tab Control") Controls_Tab."1" ("Tab Control") Controls_Tab."1" ("Tab Control") Controls_Tab."1" ("Tab Control") Controls_Tab."Analysis" ("Tab Control") Controls_Tab."2" ("Tab Control")] -> w222
                  tunnel: w232 -> [_ _ _ _ _ _ _ _ w244 _ w265 w275 w283 w293 w303 w315 w325 w335 w345]
                  tunnel: w223 -> [_ _ _ _ _ _ _ _ _ w253 _ _ _ _ _ _ _ _ _]
                  frame Default {
                  }
                  frame "1" {
                  }
                  frame "2" {
                  }
                  frame "Mean" {
                  }
                  frame "Hist" {
                  }
                  frame "Lines" {
                  }
                  frame "Analysis" {
                  }
                  frame "Error" {
                  }
                  frame "Hide Controls", "Show Controls" {
                    n118 = local read "Hide controls"() -> (w242:bool)
                    n119 = Not(x=w242) -> (.not. x?=w241:bool)
                    n120 = case shown="True" w241 {
                      tunnel: w243 -> [_ _]
                      tunnel: w244 -> [w247 w250]
                      frame True {
                        n121 = Set Menu Item Info(7:"Hide Controls" ("item tag"), 10:"Show Controls" ("item name"), 11:w247) -> ()  [unwired: 4 in, 2 out]
                      }
                      frame False {
                        n122 = Set Menu Item Info(7:"Hide Controls" ("item tag"), 10:"Hide Controls" ("item name"), 11:w250) -> ()  [unwired: 4 in, 2 out]
                      }
                    }
                    n123 = property on="Hide controls" class="Bool (strict)"("Val(Sgnl)"=w241) -> ()  [unwired: 2 in, 2 out]
                  }
                  frame "Color Table" {
                    # "Enhance Low"
                    n124 = String Subset(string=w253, offset (0)=1) -> (substring=w252:string)  [unwired: 1 in]
                    n125 = case shown="\"Enhance Low\", Default" w252 {
                      tunnel: [image_color_table_presets."enhance low" ("Value (Signaling)") image_color_table_presets."blue yellow red" ("Value (Signaling)") image_color_table_presets."BYR enhance low" ("Value (Signaling)") image_color_table_presets."white blue yellow" ("Value (Signaling)") image_color_table_presets."BWR enhance low" ("Value (Signaling)") image_color_table_presets."make a new one" ("Value (Signaling)")] -> w255
                      frame "Enhance Low", Default {
                      }
                      frame "Blue Yellow Red" {
                      }
                      frame "BYR enhance low" {
                      }
                      frame "White Blue Yellow" {
                      }
                      frame "BWR enhance low" {
                      }
                      frame "Make a new one" {
                      }
                    }
                    n126 = property on="Color table" class="Enum (strict)"("Val(Sgnl)"=w255) -> ()  [unwired: 2 in, 2 out]
                  }
                  frame "Maximize ON" {
                    n127 = local read "Maximize!!"() -> (w264:bool)
                    n128 = Not(x=w264) -> (.not. x?=w263:bool)
                    n129 = case shown="False" w263 {
                      tunnel: w265 -> [w268 w271]
                      frame True {
                        n130 = Set Menu Item Info(7:"Maximize ON" ("item tag"), 10:"Maximize OFF" ("item name"), 11:w268) -> ()  [unwired: 4 in, 2 out]
                      }
                      frame False {
                        n131 = Set Menu Item Info(7:"Maximize ON" ("item tag"), 10:"Maximize ON" ("item name"), 11:w271) -> ()  [unwired: 4 in, 2 out]
                      }
                    }
                    n132 = property on="Maximize!!" class="Bool (strict)"("Val(Sgnl)"=w263) -> ()  [unwired: 2 in, 2 out]
                  }
                  frame "Autoscale ON" {
                    n133 = local read "Autoscale"() -> (w276:bool)
                    n134 = Not(x=w276) -> (.not. x?=w274:bool)
                    n135 = case shown="False" w274 {
                      tunnel: w275 -> [w278 w281]
                      frame True {
                        n136 = Set Menu Item Info(7:"Autoscale ON" ("item tag"), 10:"Autoscale OFF" ("item name"), 11:w278) -> ()  [unwired: 4 in, 2 out]
                      }
                      frame False {
                        n137 = Set Menu Item Info(7:"Autoscale ON" ("item tag"), 10:"Autoscale ON" ("item name"), 11:w281) -> ()  [unwired: 4 in, 2 out]
                      }
                    }
                    n138 = property on="Autoscale" class="Bool (strict)"("Val(Sgnl)"=w274) -> ()  [unwired: 2 in, 2 out]
                  }
                  frame "Scale ON" {
                    n139 = local read "Scale"() -> (w284:bool)
                    n140 = Not(x=w284) -> (.not. x?=w285:bool)
                    n141 = case shown="False" w285 {
                      tunnel: w283 -> [w287 w290]
                      frame True {
                        n142 = Set Menu Item Info(7:"Scale ON" ("item tag"), 10:"Scale OFF" ("item name"), 11:w287) -> ()  [unwired: 4 in, 2 out]
                      }
                      frame False {
                        n143 = Set Menu Item Info(7:"Scale ON" ("item tag"), 10:"Scale ON" ("item name"), 11:w290) -> ()  [unwired: 4 in, 2 out]
                      }
                    }
                    n144 = property on="Scale" class="Bool (strict)"("Val(Sgnl)"=w285) -> ()  [unwired: 2 in, 2 out]
                  }
                  frame "Trigger ON" {
                    n145 = local read "Trigger"() -> (w295:bool)
                    n146 = Not(x=w295) -> (.not. x?=w294:bool)
                    n147 = case shown="True" w294 {
                      tunnel: w293 -> [w297 w300]
                      frame True {
                        n148 = Set Menu Item Info(7:"Trigger ON" ("item tag"), 10:"Trigger OFF" ("item name"), 11:w297) -> ()  [unwired: 4 in, 2 out]
                      }
                      frame False {
                        n149 = Set Menu Item Info(7:"Trigger ON" ("item tag"), 10:"Trigger ON" ("item name"), 11:w300) -> ()  [unwired: 4 in, 2 out]
                      }
                    }
                    n150 = property on="Trigger" class="Bool (strict)"("Val(Sgnl)"=w294) -> ()  [unwired: 2 in, 2 out]
                  }
                  frame "Save ON" {
                    n151 = local read "Save"() -> (w305:bool)
                    n152 = Not(x=w305) -> (.not. x?=w304:bool)
                    n153 = case shown="False" w304 {
                      tunnel: w303 -> [w307 w310]
                      frame True {
                        n154 = Set Menu Item Info(7:"Save ON" ("item tag"), 10:"Save OFF" ("item name"), 11:w307) -> ()  [unwired: 4 in, 2 out]
                      }
                      frame False {
                        n155 = Set Menu Item Info(7:"Save ON" ("item tag"), 10:"Save ON" ("item name"), 11:w310) -> ()  [unwired: 4 in, 2 out]
                      }
                    }
                    n156 = property on="Save" class="Bool (strict)"("Val(Sgnl)"=w304) -> ()  [unwired: 2 in, 2 out]
                  }
                  frame "Draw Crosshair ON" {
                    n157 = local read "draw Xhair"() -> (w313:bool)
                    n158 = Not(x=w313) -> (.not. x?=w312:bool)
                    n159 = case shown="False" w312 {
                      tunnel: w315 -> [w317 w320]
                      frame True {
                        n160 = Set Menu Item Info(7:"Draw Crosshair ON" ("item tag"), 10:"Draw Crosshair OFF" ("item name"), 11:w317) -> ()  [unwired: 4 in, 2 out]
                      }
                      frame False {
                        n161 = Set Menu Item Info(7:"Draw Crosshair ON" ("item tag"), 10:"Draw Crosshair ON" ("item name"), 11:w320) -> ()  [unwired: 4 in, 2 out]
                      }
                    }
                    n162 = property on="draw Xhair" class="Bool (strict)"("Val(Sgnl)"=w312) -> ()  [unwired: 2 in, 2 out]
                  }
                  frame "Low Pass ON" {
                    n163 = local read "LowPass"() -> (w323:bool)
                    n164 = Not(x=w323) -> (.not. x?=w322:bool)
                    n165 = case shown="True" w322 {
                      tunnel: w325 -> [w327 w330]
                      frame True {
                        n166 = Set Menu Item Info(7:"Low Pass ON" ("item tag"), 10:"Low Pass OFF" ("item name"), 11:w327) -> ()  [unwired: 4 in, 2 out]
                      }
                      frame False {
                        n167 = Set Menu Item Info(7:"Low Pass ON" ("item tag"), 10:"Low Pass ON" ("item name"), 11:w330) -> ()  [unwired: 4 in, 2 out]
                      }
                    }
                    n168 = property on="LowPass" class="Bool (strict)"("Val(Sgnl)"=w322) -> ()  [unwired: 2 in, 2 out]
                  }
                  frame "Analysis ON" {
                    n169 = local read "Analysis"() -> (w333:bool)
                    n170 = Not(x=w333) -> (.not. x?=w332:bool)
                    n171 = case shown="False" w332 {
                      tunnel: w335 -> [w337 w340]
                      frame True {
                        n172 = Set Menu Item Info(7:"Analysis ON" ("item tag"), 10:"Analysis OFF" ("item name"), 11:w337) -> ()  [unwired: 4 in, 2 out]
                      }
                      frame False {
                        n173 = Set Menu Item Info(7:"Analysis ON" ("item tag"), 10:"Analysis ON" ("item name"), 11:w340) -> ()  [unwired: 4 in, 2 out]
                      }
                    }
                    n174 = property on="Analysis" class="Bool (strict)"("Val(Sgnl)"=w332) -> ()  [unwired: 2 in, 2 out]
                  }
                  frame "Beep If Saturation ON" {
                    n175 = local read "Beep If Sat."() -> (w343:bool)
                    n176 = Not(x=w343) -> (.not. x?=w342:bool)
                    n177 = case shown="True" w342 {
                      tunnel: w345 -> [w347 w350]
                      frame True {
                        n178 = Set Menu Item Info(7:"Beep If Saturation ON" ("item tag"), 10:"Beep If Saturation OFF" ("item name"), 11:w347) -> ()  [unwired: 4 in, 2 out]
                      }
                      frame False {
                        n179 = Set Menu Item Info(7:"Beep If Saturation ON" ("item tag"), 10:"Beep If Saturation ON" ("item name"), 11:w350) -> ()  [unwired: 4 in, 2 out]
                      }
                    }
                    n180 = property on="Beep If Sat." class="Bool (strict)"("Val(Sgnl)"=w342) -> ()  [unwired: 2 in, 2 out]
                  }
                }
                n181 = property on="Tab Control" class="TabCtl (strict)"("Value"=w222) -> ()  [unwired: 2 in, 2 out]
              }
              frame "Exit" {
                n182 = local write "stop"(TRUE ("stop")) -> ()
                n183 = call "StopFGV.vi"("Command"=enum16{"set", "get", "init"}."set", "Stop"=TRUE) -> ()  [unwired: 9 in, 1 out]
              }
            }
            n184 = Equal?(x=w208, y="Exit") -> (x = y?=w212:bool)
            n185 = Select(t="Macro: Exit", s=w212, f="") -> (s? t:f=w209:string)
            n186 = call <vilib>:"Add State(s) to Queue__JKI_lib_State_Machine.vi"("State(s) in Front (\"\")"=w209, "State(s) in (\"\")"=w216) -> ("States Out"=w215:string)  [unwired: 13 in]
          }
          event "Maximize!!": Value Change {
            n187 = event-data() -> ()  [unwired: 1 in, 6 out]
            n188 = property class="VI"(error in=w358) -> (error out=w360:errorcluster, "Front Panel.PanelBounds"=w361:T7)  [unwired: 1 in, 1 out]
            n189 = case shown="False" "Maximize!!" {
              tunnel: w361 -> [w366 w370]
              tunnel: [w366 w370] -> _
              tunnel: [w363 w369] -> w357
              tunnel: w360 -> [w364 w367]
              frame False {
                n190 = property class="VI"(error in=w364, "Front Panel Window:State"=T9."Standard") -> (error out=w363:errorcluster)  [unwired: 1 in, 1 out]
              }
              frame True {
                n191 = property class="VI"(error in=w367, "Front Panel Window:State"=T9."Maximized") -> (error out=w369:errorcluster)  [unwired: 1 in, 1 out]
                n192 = Wait (ms)(milliseconds to wait=u32 200) -> ()  [unwired: 1 out]
              }
            }
            n193 = call <vilib>:"Add State(s) to Queue__JKI_lib_State_Machine.vi"("State(s) in (\"\")"=w356) -> ("States Out"=w355:string)  [unwired: 14 in]
          }
          event "Fit Control": Value Change {
            n194 = event-data() -> ()  [unwired: 1 in, 6 out]
            n195 = invoke on="Image (IMAQ)" class="ImageControl" method="FitControlToPane"(error in=w373) -> (error out=w372:errorcluster)  [unwired: 2 in, 2 out]
          }
        }
      }
      frame "---------- Core ----------" {
        # "Do not put any code in this frame.\n(it is a separator no-op)"
        n196 = call <vilib>:"Add State(s) to Queue__jki_lib_state_machine.vi"("State(s) in (\"\")"=w379) -> ("States Out"=w378:string)  [unwired: 14 in]
      }
      frame Default {
        w389 = 42 items=["No error", "Argument error", "Memory is full", "Out of zone", "End of file", "File already open", "Generic file I/O error", "File not found", "File permission error", "Disk is full", "Duplicate path", "Too many files open", "System feature not enabled", "Resource file not found", "Cannot add resource", "Resource not found", "Image not found", "Image memory error", "Pen does not exist", "Config type invalid", "Config token not found", "Config parse error", "Config memory error", "Bad external code format", "Bad external code offset", "External code not present", "Null window", "Destroy window error", "Null menu", "Print aborted", "Bad print record", "Print driver error", "Windows error during printing", "Memory error during printing", "Print dialog error", "Generic print error", "Invalid device refnum", "Device not found", "Device parameter error", "Device unit error", "Cannot open device", "Device call aborted", "Generic error", "Cancelled by user", "Object ID too low", "Object ID too high", "Object not in heap", "Unknown heap", "Unknown object (invalid DefProc)", "Unknown object (DefProc not in table)", "Message out of range", "Invalid (null) method", "Unknown message", "Manager call not supported", "Bad address", "Network operation in progress", "Network operation timed out", "Connection is busy", "Network attribute not supported", "Network error", "Address in use", "System out of memory", "Connection aborted", "Connection refused", "Not connected", "Already connected", "Connection closed", "Initialization error (interapplication manager)", "Bad occurrence", "Wait on unbound occurrence handler", "Occurrence queue overflow", "Datalog type conflict", "Unused", "Unrecognized type (interapplication manager)", "Memory corrupt", "Failed to make temporary DLL", "Old CIN version", "Drag socket not found", "Failed to load drop-object", "Failed to register OLE object", "Failed to release OLE object", "Format specifier type mismatch", "Unknown format specifier", "Too few format specifiers", "Too many format specifiers", "Scan failed", "Newer CIN version", "Error converting to variant", "Runtime menu error", "Password tampered", "Variant attribute not found", "Incompatible variant data type", "Event data is not available", "Event Store is not present", "Occurrence is not found", "Event Queue is not created", "Event info is not available", "Refnum passed is NULL", "Error retrieving Class GUID", "Error retrieving CoClass GUID", "Error retrieving TypeLib GUID.", "Bad built application magic bytes.", "Specific driver is different from the specific driver associated with the Logical Name.", "There is no session opened to the class driver.", "Max Error", "MAX - Error with config objects", "MAX - Error loading configuration", "MAX - Group not supported"]
        # "Current State"
        # "Do not delete, rename, or modify this frame.\n(this is used to capture unhandled states and typos)"
        # "Handle mistyped state name (developer tool)"
        n197 = Format Into String(format string="Software Exception: Unhandled State \"%s\"." ("message"), error in=w385, w380) -> (resulting string=w388:string, error out=w387:errorcluster)  [unwired: 1 in]
        n198 = call <vilib>:"Error Cluster From Error Code.vi"("show call chain? (False)"=TRUE, "error in (no error)"=w387, "error message (\"\")"=w388, "error code (0)"=w389) -> ("error out"=w386:errorcluster)  [unwired: 5 in]
        n199 = call <vilib>:"Add State(s) to Queue__jki_lib_state_machine.vi"("State(s) in (\"\")"=w384) -> ("States Out"=w383:string)  [unwired: 14 in]
      }
      frame "Initialize Core Data" {
        # "Do not delete, rename, or modify this frame.\n(this is used to determine panel behavior on exit)"
        # "originally closed?"
        # "exe?"
        # "If panel starts closed or is an EXE, then close it when we exit"
        n200 = property class="VI"() -> ("Front Panel.Open"=w398:bool)  [unwired: 2 in, 2 out]
        n201 = property class="App"() -> ("App.Kind"=w397:T10)  [unwired: 2 in, 2 out]
        n202 = control-ref of="Current VI Reference"() -> (w391:refnum<vi>)
        n203 = Not(x=w398) -> (.not. x?=w395:bool)
        n204 = Equal?(x=w397, y=T10."Run Time System" ("Application:Kind")) -> (x = y?=w394:bool)
        n205 = Or(x=w395, y=w394) -> (x .or. y?=w392:bool)
        n206 = Bundle By Name(cluster=w393, "Core.Current VI Reference"=w391, "Core.Close Panel on Exit?"=w392) -> (w400:T15)
        n207 = call <vilib>:"Add State(s) to Queue__jki_lib_state_machine.vi"("State(s) in (\"\")"=w402) -> ("States Out"=w401:string)  [unwired: 14 in]
      }
      frame "Error Handler" {
        # "Unhandled Error -- Display it"
        # "Handle any errors here.\nYou can also output any states to clean-up after errors occur"
        # "Clear error"
        n208 = call <vilib>:"General Error Handler.vi"("error in (no error)"=w404) -> ()  [unwired: 10 in, 5 out]
        n209 = call <vilib>:"Add State(s) to Queue__jki_lib_state_machine.vi"("State(s) in Front (\"\")"="/* Post Error States", "State(s) in (\"\")"=w408) -> ("States Out"=w407:string)  [unwired: 13 in]
      }
      frame "Exit" {
        # "Do not put any code in this frame.\n(No errors that occur here will be handled.)"
        n210 = call <vilib>:"Add State(s) to Queue__jki_lib_state_machine.vi"("State(s) in (\"\")"=w413) -> ("States Out"=w412:string)  [unwired: 14 in]
      }
      frame "---------- Data ----------" {
        # "Do not put any code in this frame.\n(It is a separator no-op. You can make a copy of this frame to create a new Data frame)"
        n211 = call <vilib>:"Add State(s) to Queue__jki_lib_state_machine.vi"("State(s) in (\"\")"=w417) -> ("States Out"=w416:string)  [unwired: 14 in]
      }
      frame "Data: Initialize" {
        w418 = T14 {"Port"=0, "Remote Host"="", "All Devices"=[], "New Device"=FALSE}  # TCP Cluster
        w419 = T13 {"Color table"=enum."enhance low", "Button Label"=""}  # IMG Features
        w422 = T16 0 items=["Grayscale (U8)", "Grayscale (I16)", "Grayscale (SGL)", "Complex (CSG)", "RGB (U32)", "HSL (U32)", "RGB (U64)", "Grayscale (U16)"] ("Image Type")
        w423 = string[] []  # subscribe messages
        w425 = T12 {"Image Out"=refnum, "valid image"=FALSE, "X resolution"=0, "Y resolution"=0, "Image Area"={"Width"=0, "Height"=0}, "zoom to fit"=FALSE, "Image Center"={"X"=0, "Y"=0}, "Max count"=0.0}  # Image Data
        w428 = T17 {"Current VI Reference"=refnum, "Close Panel on Exit?"=FALSE}  # Core
        # "Initialize the shift-register data, here.\n(data names are defined by what you wire into the bundle function)"
        n212 = call "IMAQ Create"("Image Name"="image out", "Image Type"=w422) -> ("New Image"=w420:T2)  [unwired: 3 in, 1 out]
        n213 = Bundle By Name(cluster=w425, "Image Out"=w420) -> (w424:T12)
        n214 = Bundle("Core"=w428, "tcp connections"=refnum<k5>[] [], "subscribe messages"=w423, "Image Data"=w424, "images"=T2[] [], "IMG Features"=w419, "TCP Cluster"=w418) -> (w430:T15)  [unwired: 1 in]
        n215 = call <vilib>:"Add State(s) to Queue__jki_lib_state_machine.vi"("State(s) in (\"\")"=w432) -> ("States Out"=w431:string)  [unwired: 14 in]
      }
      frame "Data: Cleanup" {
        # "Cleanup any data and references, here.\n(this is called automatically, by the Macro: Exit)"
        n216 = Unbundle By Name(w444) -> ("Core.Current VI Reference"=w445:refnum<vi>, "tcp connections"=w443:refnum<k5>[], "Image Data.Image Out"=w441:T2, "images"=w440:T2[])
        n217 = Index Array(array=w440) -> (element=w438:T2)  [unwired: 1 in]
        n218 = Index Array(array=w443) -> (element=w442:refnum<k5>)  [unwired: 1 in]
        n219 = TCP Close Connection(connection ID=w442, error in (no error)=w436) -> (error out=w439:errorcluster)  [unwired: 1 in, 1 out]
        n220 = call "IMAQ Dispose"("Image"=w441, "error in (no error)"=w439) -> ("error out"=w437:errorcluster)  [unwired: 4 in]
        n221 = call "IMAQ Dispose"("Image"=w438, "error in (no error)"=w437) -> ("error out"=w435:errorcluster)  [unwired: 4 in]
        n222 = Close Reference(reference=w445, error in (no error)=w435) -> (error out=w434:errorcluster)
        n223 = call <vilib>:"Clear Errors.vi"("error in (no error)"=w434) -> ("error out"=w433:errorcluster)  [unwired: 6 in]
        n224 = call <vilib>:"Add State(s) to Queue__jki_lib_state_machine.vi"("State(s) in (\"\")"=w447) -> ("States Out"=w446:string)  [unwired: 14 in]
      }
      frame "---------- UI ----------" {
        # "Do not put any code in this frame.\n(It is a separator no-op. You can make a copy of this frame to create a new UI frame)"
        n225 = call <vilib>:"Add State(s) to Queue__jki_lib_state_machine.vi"("State(s) in (\"\")"=w451) -> ("States Out"=w450:string)  [unwired: 14 in]
      }
      frame "UI: Initialize" {
        w452 = FALSE ("hide controls")
        w456 = u32 3 items=["Grayscale", "Binary", "Gradient", "Rainbow", "Temperature", "User Defined"] ("Palette:Palette Type")
        # "Initialize the User Interface, here.\n(this is called automatically, by the Macro: Init)"
        n226 = property on="Scale" class="Bool (strict)"("Value"=w452) -> ()  [unwired: 2 in, 2 out]
        n227 = property on="Analysis" class="Bool (strict)"("Value"=w452) -> ()  [unwired: 2 in, 2 out]
        n228 = property on="Autoscale" class="Bool (strict)"("Value"=w452) -> ()  [unwired: 2 in, 2 out]
        n229 = property on="Beep If Sat." class="Bool (strict)"("Value"=w452) -> ()  [unwired: 2 in, 2 out]
        n230 = property on="Maximize!!" class="Bool (strict)"("Value"=w452) -> ()  [unwired: 2 in, 2 out]
        n231 = local write "Image (IMAQ)"(T2 refnum ("Image Out")) -> ()
        n232 = local write "Hide controls"(FALSE ("hide controls")) -> ()
        n233 = property on="Splitter" class="Splitter"("Position"=372 ("Splitter Position")) -> ()  [unwired: 2 in, 2 out]
        n234 = property on="Image (IMAQ)" class="ImageControl"("Palette Type"=w456) -> ()  [unwired: 2 in, 2 out]
        n235 = property on="LowPass" class="Bool (strict)"("Value"=w452) -> ()  [unwired: 2 in, 2 out]
        n236 = property on="Hide controls" class="Bool (strict)"("Value"=w452) -> ()  [unwired: 2 in, 2 out]
        n237 = property on="draw Xhair" class="Bool (strict)"("Value"=w452) -> ()  [unwired: 2 in, 2 out]
        n238 = property on="Save" class="Bool (strict)"("Value"=w452) -> ()  [unwired: 2 in, 2 out]
        n239 = property on="Trigger" class="Bool (strict)"("Value"=w452) -> ()  [unwired: 2 in, 2 out]
        n240 = Bundle By Name(cluster=w455, "Image Data.zoom to fit"=TRUE) -> (w454:T15)
        n241 = call <vilib>:"Add State(s) to Queue__jki_lib_state_machine.vi"("State(s) in (\"\")"=w462) -> ("States Out"=w461:string)  [unwired: 14 in]
      }
      frame "UI: Get Devices" {
        n242 = control-ref of="This VI"() -> (w473:refnum<vi>)
        n243 = call "getPortAndIP.vi"("Device Name"=w469, "This Vi"=w473) -> ("Remote Host"=w463:string, "port or service name"=w464:u16, "reference out"=w472:refnum<vi>)  [unwired: 2 in, 2 out]
        "port or service name" <- w464
        "Remote Host" <- w463
        n244 = property class="VI"(reference=w472, "Front Panel.Resizeable"=TRUE ("Front Panel Window:Resizable")) -> ()  [unwired: 1 in, 2 out]
        n245 = call "ConnectionFGV.vi"("command"=enum16{"get", "set", "init"}."set", "Remote Host in"=w463, "port or service name in"=w464) -> ()  [unwired: 7 in, 2 out]
        n246 = Bundle By Name(cluster=w466, "TCP Cluster.Port"=w464, "TCP Cluster.Remote Host"=w463) -> (w465:T15)
        "Device Name (h)" <- w469
        "Left" <- w467
        "Top" <- w468
      }
      frame "UI: Update Devices" {
        w483 = "fixsize" ("item tag")
        n247 = Current VI's Menubar() -> (w485:refnum<k9>)
        n248 = for {
          tunnel: [w490] -> w476 mode=concatenating
          tunnel: string[] ["Photometrics_CH-250_Cam", "Point Grey Camera", "Photometrics Cam", "Manta Camera", "Basler Camera", "AndorCamera", "SVimage"] -> [w489] mode=indexing
          n249 = call "getDevices.vi"("Device Class"=w489) -> ("All Devices"=w490:string[])
        }
        n250 = Get Menu Item Info(7:"ratio" ("item tag"), 11:w485) -> (3:w482:refnum<k9>)  [unwired: 1 in, 6 out]
        n251 = Set Menu Item Info(7:w483, 9:TRUE ("enabled"), 11:w482) -> (3:w481:refnum<k9>)  [unwired: 4 in, 1 out]
        n252 = for {
          tunnel: w481 -> [w498]
          tunnel: [w497] -> w484
          tunnel: w476 -> [w495] mode=indexing
          n253 = Insert Menu Items(5:"Devices" ("menu tag"), 7:w495, 8:w495, 9:w498) -> (3:w497:refnum<k9>)  [unwired: 2 in, 2 out]
        }
        n254 = disable-structure shown="Disabled" {
          disable-tunnel: [w493 TRUE] -> _
          disable-tunnel: w483 -> [w492 _]
          disable-tunnel: w482 -> [w491 _]
          frame Disabled {
            n255 = Get Menu Item Info(7:w492, 11:w491) -> (4:w493:bool)  [unwired: 1 in, 6 out]
          }
          frame Enabled {
          }
        }
        n256 = Bundle By Name(cluster=w478, "TCP Cluster.All Devices"=w476) -> (w477:T15)
        n257 = Enable Menu Tracking(4:w484) -> ()  [unwired: 2 in, 2 out]
      }
      frame "UI: Hidden Devices" {
        n258 = Unbundle By Name(w500) -> ("TCP Cluster.Port"=w499:u16)
        n259 = call "connectUDP.vi"("port or service name NOT USED"=w499) -> ("fast ID (h)"=→"fast ID (h)":refnum<k16>, "slow ID (h)"=→"slow ID (h)":refnum<k16>, "connections (hidden)"=→"connections (hidden)":variant[], "local Port"=→"local Port":u16)
      }
      frame "UI: Cursor Set" {
        # "Argument"
        # "Set and Unset Cursor Busy.\n(Usage: \"UI: Cursor Set >> Busy|Idle\")"
        n260 = case shown="\"Idle\", Default" w507 {
          tunnel: w509 -> [w514 w516]
          tunnel: [w513 w515] -> w508
          frame "Idle", Default {
            n261 = call <vilib>:"Unset Busy.vi"("error in (no error)"=w514) -> ("error out"=w513:errorcluster)  [unwired: 10 in]
          }
          frame "Busy" {
            n262 = call <vilib>:"Set Busy.vi"("error in (no error)"=w516) -> ("error out"=w515:errorcluster)  [unwired: 9 in, 1 out]
          }
        }
        n263 = call <vilib>:"Add State(s) to Queue__jki_lib_state_machine.vi"("State(s) in (\"\")"=w512) -> ("States Out"=w511:string)  [unwired: 14 in]
      }
      frame "UI: Front Panel State" {
        # "Argument"
        # "Set Front Panel Open or Closed\n(Usage: \"UI: Front Panel State >> Open|Close\")"
        n264 = Unbundle By Name(w519) -> ("Core.Current VI Reference"=w518:refnum<vi>)
        n265 = case shown="\"Open\", Default" w517 {
          tunnel: w521 -> [w527 w540]
          tunnel: [w529 w541] -> w520
          tunnel: w518 -> [w528 w538]
          frame "Open", Default {
            n266 = property class="VI"(reference=w528, error in=w527) -> (reference out=w525:refnum<vi>, error out=w526:errorcluster, "Front Panel.Open"=w524:bool)
            n267 = case shown="True" w524 {
              tunnel: [w532 w535] -> w529
              tunnel: w526 -> [w531 w535]
              tunnel: w525 -> [w530 _]
              frame False {
                n268 = invoke class="VI" method="FP.Open"(reference=w530, error in=w531, "Activate"=TRUE, "State"=T9."Standard") -> (error out=w532:errorcluster)  [unwired: 1 in, 4 out]
              }
              frame True {
              }
            }
          }
          frame "Close" {
            n269 = property class="VI"(reference=w538, error in=w540) -> (reference out=w537:refnum<vi>, error out=w539:errorcluster, "Front Panel.Open"=w536:bool)
            n270 = case shown="True" w536 {
              tunnel: [w542 w545] -> w541
              tunnel: w539 -> [w542 w544]
              tunnel: w537 -> [_ w543]
              frame False {
              }
              frame True {
                n271 = invoke class="VI" method="FP.Close"(reference=w543, error in=w544) -> (error out=w545:errorcluster)  [unwired: 1 in, 2 out]
              }
            }
          }
        }
        n272 = call <vilib>:"Add State(s) to Queue__jki_lib_state_machine.vi"("State(s) in (\"\")"=w523) -> ("States Out"=w522:string)  [unwired: 14 in]
      }
      frame "---------- Macro ----------" {
        # "Do not put any code in this frame.\n(It is a separator no-op. You can make a copy of this frame to create a new Macro frame)"
        n273 = call <vilib>:"Add State(s) to Queue__jki_lib_state_machine.vi"("State(s) in (\"\")"=w549) -> ("States Out"=w548:string)  [unwired: 14 in]
      }
      frame "Macro: Initialize" {
        w550 = "Data: Initialize\nInitialize Core Data\nUI: Initialize\nUI: Front Panel State >> Open"  # Data: Initialize Initialize Core Data UI: Initialize UI: Front Panel State >> Open
        # "Initialization Macro\n(This is called once, when the VI starts)"
        n274 = call <vilib>:"Add State(s) to Queue__jki_lib_state_machine.vi"("State(s) in Front (\"\")"=w550, "State(s) in (\"\")"=w554) -> ("States Out"=w553:string)  [unwired: 13 in]
      }
      frame "Macro: valid image" {
        # "Initialization Macro\n(This is called once, when the VI starts)"
        n275 = call <vilib>:"Add State(s) to Queue__jki_lib_state_machine.vi"("State(s) in Front (\"\")"="Action: Get Image\nAction: Get Image Size\nAction: Resize FP\nAction: Set Zoom Factor", "State(s) in (\"\")"=w559) -> ("States Out"=w558:string)  [unwired: 13 in]
      }
      frame "Macro: Exit" {
        # "Exit Macro\n(This is called once, when the VI exits)"
        n276 = Unbundle By Name(w566) -> ("Core.Close Panel on Exit?"=w565:bool)
        n277 = Select(t="UI: Front Panel State >> Close", s=w565, f="") -> (s? t:f=w562:string)
        n278 = call <vilib>:"Add State(s) to Queue__jki_lib_state_machine.vi"("State(s) in (\"\")"=w562, "State(s) at Back (\"\")"="Data: Cleanup\nExit") -> ("States Out"=w560:string)  [unwired: 13 in]
        n279 = call <vilib>:"Add State(s) to Queue__jki_lib_state_machine.vi"("State(s) in Front (\"\")"=w560, "State(s) in (\"\")"=w569) -> ("States Out"=w568:string)  [unwired: 13 in]
      }
      frame "---------- New Category ----------" {
        # "Template Separator\n(You can make a copy of, or modify, this frame)"
        n280 = call <vilib>:"Add State(s) to Queue__jki_lib_state_machine.vi"("State(s) in (\"\")"=w573) -> ("States Out"=w572:string)  [unwired: 14 in]
      }
      frame "Action: open tcp" {
        # "will probably delete this"
        n281 = Build Array("String") -> (w579:string[])
        n282 = call "open tcp connections and create images.vi"("devices to get data from"=w579) -> ("images"=w575:T2[], "subscribe messages\nfor process vis"=w574:string[], "tcp connections"=w576:refnum<k5>[])  [unwired: 8 in]
        n283 = Bundle By Name(cluster=w578, "tcp connections"=w576, "subscribe messages"=w574, "images"=w575) -> (w577:T15)
        n284 = call <vilib>:"Add State(s) to Queue__jki_lib_state_machine.vi"("State(s) in (\"\")"=w583) -> ("States Out"=w582:string)  [unwired: 14 in]
      }
      frame "Action: Get Image" {
        w588 = 255.0  # A
        w601 = 5.0  # No spot sizes 2
        w600 = 15.0  # w
        w605 = T16 0 items=["Grayscale (U8)", "Grayscale (I16)", "Grayscale (SGL)", "Complex (CSG)", "RGB (U32)", "HSL (U32)", "RGB (U64)", "Grayscale (U16)"] ("Image Type")
        n285 = Random Number (0-1)() -> (number: 0 to 1=w589:dbl)
        n286 = Multiply(x=w601, y=w600) -> (x*y=w602:dbl)
        n287 = Add(x=0.5, y=w589) -> (x+y=w591:dbl)
        n288 = Random Number (0-1)() -> (number: 0 to 1=w596:dbl)
        n289 = Multiply(x=w588, y=w591) -> (x*y=w587:dbl)
        n290 = Divide(x=w602, y=2.0) -> (x/y=w593:dbl)
        n291 = Initialize Array(0.0 ("element"), w602, w602) -> (w599:dbl[][])
        n292 = Add(x=0.5, y=w596) -> (x+y=w594:dbl)
        n293 = Multiply(x=w593, y=w594) -> (x*y=w592:dbl)
        n294 = for {
          tunnel: w599 -> [w616] mode=indexing
          shift-right: [w614] -> w597
          shift-left: w599 -> [w615]
          tunnel: w587 -> [w613]
          tunnel: w593 -> [w611]
          tunnel: w600 -> [w610]
          tunnel: w592 -> [w609]
          i -> [w612]
          n295 = for {
            tunnel: w616 -> [_] mode=indexing
            shift-right: [w625] -> w614
            shift-left: w615 -> [w626]
            tunnel: w612 -> [w624]
            tunnel: w613 -> [w621]
            tunnel: w612 -> [w620]
            tunnel: w611 -> [w619]
            tunnel: w610 -> [w618]
            tunnel: w609 -> [w617]
            i -> [w623]
            n296 = formula code="I=A*exp((-2/w**2)*((y-x0)**2+(x-y0)**2));"("y"=w623, "A"=w621, "x0"=w619, "x"=w620, "w"=w618, "y0"=w617) -> ("I"=w622:dbl)
            n297 = Replace Array Subset(array=w626, new element=w622, index (row)=w624, index (col)=w623) -> (w625:dbl[][])
          }
        }
        n298 = call "IMAQ Create"("Image Name"="ddfgd", "Image Type"=w605) -> ("New Image"=w604:T2)  [unwired: 3 in, 1 out]
        n299 = call "IMAQ ArrayToImage"("Image Pixels (U8)"=w597, "Image"=w604) -> ("Image Out"=w584:T2)  [unwired: 8 in, 1 out]
        "image::1" <- w584
        n300 = Bundle By Name(cluster=w586, "Image Data.Image Out"=w584) -> (w585:T15)
      }
      frame "Action: Wait TCP" {
        n301 = call "WaitFGV.vi"("Command"=enum16{"get", "set", "init"}."set", "milliseconds to wait"="time to wait (TCP)") -> ()  [unwired: 9 in, 1 out]
      }
      frame "Action: Load Image" {
        # "Load Image from File"
        n302 = Unbundle By Name(w633) -> ("Image Data.zoom to fit"=w632:bool)
        n303 = disable-structure shown="Enabled" {
          disable-tunnel: w636 -> [w641 _]
          frame Disabled {
            n304 = property on="Splitter" class="Splitter"(error in=w641, "Position"=372 ("Splitter Position")) -> ()  [unwired: 1 in, 2 out]
          }
          frame Enabled {
          }
        }
        n305 = property on="Image (IMAQ)" class="ImageControl"("Zoom to Fit Mode"=w632) -> ()  [unwired: 2 in, 2 out]
        n306 = disable-structure shown="Enabled" {
          disable-tunnel: [_ w643] -> w635
          disable-tunnel: w636 -> [_ w646]
          disable-tunnel: [_ w644] -> w637
          disable-tunnel: w633 -> [_ w645]
          frame Disabled {
          }
          frame Enabled {
            n307 = disable-structure shown="Enabled" {
              disable-tunnel: w646 -> [w652 w659]
              disable-tunnel: w645 -> [w651 w655]
              disable-tunnel: [w650 w656] -> w644
              disable-tunnel: [_ w658] -> w643
              frame Disabled {
                n308 = Unbundle By Name(w651) -> ("tcp connections"=w649:refnum<k5>[], "subscribe messages"=w648:string[], "images"=w647:T2[])
                n309 = call "get multiple images over tcp.vi"("ErrorIn"=w652, "images In"=w647, "subscribeMessages"=w648, "TCP_Refs In"=w649) -> ("Images out"=w653:T2[])  [unwired: 3 in, 4 out]
                n310 = Index Array(array=w653) -> (element=w650:T2)  [unwired: 1 in]
              }
              frame Enabled {
                n311 = Unbundle By Name(w655) -> ("Image Data.Image Out"=w657:T2, "Image Data.Image Out"=w654:T2)
                n312 = call "IMAQ Copy"("error in (no error)"=w659, "Image Dst"=w657, "Image Src"=w654) -> ("error out"=w658:errorcluster, "Image Dst Out"=w656:T2)  [unwired: 3 in]
              }
            }
          }
        }
        n313 = Bundle By Name(cluster=w633, "Image Data.Image Out"=w637) -> (w638:T15)
        n314 = call <vilib>:"Add State(s) to Queue__jki_lib_state_machine.vi"("State(s) in Front (\"\")"="Action: Get Image Size" ("State(s) in Front (\"\")"), "State(s) in (\"\")"=w640) -> ("States Out"=w639:string)  [unwired: 13 in]
      }
      frame "Action: Get Image Size" {
        # "Set IMAQ control size to \nImage size (x and y resolution)"
        n315 = Unbundle By Name(w671) -> ("Image Data.X resolution"=w673:i32, "Image Data.Y resolution"=w672:i32, "Image Data.Image Out"=w661:T2)
        "Image (IMAQ)" <- w661
        n316 = case shown="No Error" w666 {
          selector: w666 -> [w680 w697]
          tunnel: [w681 _] -> w669
          tunnel: [w678 _] -> w668
          tunnel: w661 -> [w679 _]
          tunnel: [w688 _] -> w667
          tunnel: [w687 w697] -> w665
          tunnel: [w676 _] -> w662
          tunnel: w673 -> [w685 _]
          tunnel: w672 -> [w684 _]
          tunnel: [w675 FALSE ("valid Image")] -> w660
          frame No Error {
            n317 = call "Get Resolution.vi"("Image"=w679, "error in (no error)"=w680) -> ("X Resolution"=w681:i32, "Y Resolution"=w678:i32, "Image Area:Size:All Elements"=w688:cluster{"Width":u32, "Height":u32}, "valid Image"=w675:bool, "error out"=w686:errorcluster)  [unwired: 9 in]
            n318 = Build Array(w685, w684) -> (w683:i32[])
            n319 = Build Array(w681, w678) -> (w682:i32[])
            n320 = Not Equal?(x=w683, y=w682) -> (x != y?=w677:bool)
            n321 = And(x=w677, y=w675) -> (x .and. y?=w674:bool)
            n322 = case shown="True" w674 {
              tunnel: w688 -> [_ _]
              tunnel: [w690 w693] -> w687
              tunnel: w686 -> [w690 w691]
              tunnel: ["" "Macro: valid image" ("State(s) in Front (\"\")")] -> w676
              frame False {
                (unwired) FALSE
              }
              frame True {
                n323 = disable-structure shown="Enabled" {
                  disable-tunnel: w691 -> [w695 _]
                  disable-tunnel: [w694 _] -> w693
                  frame Enabled {
                    n324 = invoke on="Image (IMAQ)" class="ImageControl" method="FitControlToPane"(error in=w695) -> (error out=w694:errorcluster)  [unwired: 2 in, 2 out]
                  }
                  frame Disabled {
                  }
                }
              }
            }
          }
          frame Error {
          }
        }
        n325 = Bundle By Name(cluster=w671, "Image Data.valid image"=w660, "Image Data.X resolution"=w669, "Image Data.Y resolution"=w668, "Image Data.Image Area"=w667) -> (w670:T15)
        n326 = call <vilib>:"Add State(s) to Queue__jki_lib_state_machine.vi"("State(s) in Front (\"\")"=w662, "State(s) in (\"\")"=w664) -> ("States Out"=w663:string)  [unwired: 13 in]
      }
      frame "Action: Resize FP" {
        # "Resize FP as per\nthe image size"
        # "Adjust the aspect ration as per the \nresize image height and width"
        # "Aspect ratio"
        # "Resizes Front panel as per the image size"
        n327 = disable-structure shown="Enabled" {
          disable-tunnel: w716 -> [w720 _]
          disable-tunnel: [w719 _] -> w699
          frame Enabled {
            n328 = invoke on="Image (IMAQ)" class="ImageControl" method="FitControlToPane"(error in=w720) -> (error out=w719:errorcluster)  [unwired: 2 in, 2 out]
          }
          frame Disabled {
          }
        }
        n329 = Unbundle By Name(w718) -> ("Image Data.Y resolution"=w701:i32, "Image Data.X resolution"=w700:i32)
        n330 = property on="Image (IMAQ)" class="ImageControl"(error in=w699) -> (error out=w703:errorcluster, "Image Area Height"=w714:u32, "Image Area Width"=w711:u32)  [unwired: 1 in, 1 out]
        n331 = Divide(x=w701, y=w700) -> (x/y=w715:dbl)
        n332 = control-ref of="This VI"() -> (w710:refnum<vi>)
        n333 = property class="VI"(reference=w710, error in=w703) -> (reference out=w707:refnum<vi>, error out=w702:errorcluster, "Front Panel.PanelBounds"=w708:T7)
        n334 = Divide(x=w714, y=w715) -> (x/y=w712:dbl)
        n335 = Subtract(x=w712, y=w711) -> (x-y=w713:dbl)
        n336 = Unbundle By Name(w708) -> ("Right"=w706:i16)
        n337 = To Word Integer(number=w713) -> (16bit integer=w705:i16)
        n338 = Add(x=w706, y=w705) -> (x+y=w704:i16)
        n339 = Bundle By Name(cluster=w708, "Right"=w704) -> (w709:T7)
        n340 = property class="VI"(reference=w707, error in=w702, "Front Panel.PanelBounds"=w709) -> (error out=w717:errorcluster)  [unwired: 1 out]
      }
      frame "Action: Set Zoom Factor" {
        # "Changed size of image"
        # "Calcultes zoom factor for image as per the changed size of image"
        n341 = Unbundle By Name(w728) -> ("Image Data.Image Area"=w730:cluster{"Width":u32, "Height":u32}, "Image Data.Image Center"=w725:cluster{"X":u32, "Y":u32}, "Image Data.zoom to fit"=w724:bool)
        n342 = disable-structure shown="Enabled" {
          disable-tunnel: w723 -> [w737 _]
          disable-tunnel: [w736 _] -> w722
          frame Enabled {
            n343 = invoke on="Image (IMAQ)" class="ImageControl" method="FitControlToPane"(error in=w737) -> (error out=w736:errorcluster)  [unwired: 2 in, 2 out]
          }
          frame Disabled {
          }
        }
        n344 = property on="Image (IMAQ)" class="ImageControl"(error in=w722) -> ("Image Area Size"=w734:cluster{"Width":u32, "Height":u32})  [unwired: 1 in, 2 out]
        n345 = Not Equal?(x=w730, y=w734) -> (x != y?=w735:bool)
        n346 = case shown="True" w735 {
          tunnel: w734 -> [_ w744]
          tunnel: w730 -> [_ w743]
          tunnel: [_ w739] -> w733
          frame False {
          }
          frame True {
            n347 = property on="Image (IMAQ)" class="ImageControl"() -> ("ZoomSingle"=w742:cluster{"X":sgl, "Y":sgl})  [unwired: 2 in, 2 out]
            n348 = Divide(x=w744, y=w743) -> (x/y=w740:cluster{"Width":dbl, "Height":dbl})
            n349 = Unbundle(w740) -> ("Height"=w738:dbl)  [unwired: 1 out]
            n350 = Multiply(x=w738, y=w742) -> (x*y=w741:cluster{"X":dbl, "Y":dbl})
            n351 = property on="Image (IMAQ)" class="ImageControl"("ZoomSingle"=w741) -> (error out=w739:errorcluster)  [unwired: 2 in, 1 out]
          }
        }
        n352 = property on="Image (IMAQ)" class="ImageControl"(error in=w733, "Image Center Position"=w725) -> (error out=w731:errorcluster)  [unwired: 1 in, 1 out]
        n353 = property on="Image (IMAQ)" class="ImageControl"(error in=w731, "Zoom to Fit Mode"=w724) -> (error out=w732:errorcluster)  [unwired: 1 in, 1 out]
        n354 = property on="Image (IMAQ)" class="ImageControl"(error in=w732) -> (error out=w729:errorcluster, "Image Area Size"=w726:cluster{"Width":u32, "Height":u32})  [unwired: 1 in, 1 out]
        n355 = Bundle By Name(cluster=w728, "Image Data.Image Area"=w726) -> (w727:T15)
      }
      frame "Action: Color Table" {
        w749 = u32 5 items=["Grayscale", "Binary", "Gradient", "Rainbow", "Temperature", "User Defined"] ("Palette:Palette Type")
        # "IMAQ color table presets"
        n356 = Unbundle By Name(w748) -> ("IMG Features.Color table"=w747:T1)
        n357 = call "IMAQ color table presets.vi"("Color table"=w747) -> ("Array"=w746:cluster{"R":u8, "G":u8, "B":u8}[])  [unwired: 10 in]
        n358 = property on="Image (IMAQ)" class="ImageControl"("Palette Type"=w749, "User Palette"=w746) -> ()  [unwired: 2 in, 2 out]
      }
      frame "Action: Draw Crosshair IMAQ" {
        n359 = Unbundle By Name(w760) -> ("Image Data.Image Out"=w758:T2)
        n360 = case shown="False" "draw Xhair" {
          tunnel: "Target.Y" -> [_ w774]
          tunnel: "Target.X" -> [_ w775]
          tunnel: w758 -> [w770 w778]
          tunnel: [w769 w776] -> w751
          tunnel: T11 {"Left"=0, "Top"=0, "Right"=0, "Bottom"=0} ("Bounding Rectangle") -> [_ w777]
          tunnel: w756 -> [w765 w772]
          tunnel: [w764 w771] -> w757
          frame False {
            n361 = Build Array("donotrename" ("String")) -> (w766:string[])
            n362 = call "IMAQ Clear Overlay"("Groups"=w766, "error in (no error)"=w765, "Image"=w770) -> ("error out"=w768:errorcluster, "Image Out"=w769:T2)  [unwired: 7 in]
            n363 = call <vilib>:"Clear Errors.vi"("error in (no error)"=w768) -> ("error out"=w764:errorcluster)  [unwired: 6 in]
          }
          frame True {
            n364 = call "draw crosshair imaq.vi"("Target.Y"=w774, "size"="size 2", "error in (no error)"=w772, "Target.X"=w775, "Bounding Rectangle"=w777, "image in"=w778) -> ("error out"=w771:errorcluster, "image out"=w776:T2)  [unwired: 4 in]
          }
        }
        n365 = Bundle("Target.X"="Target.X", "Target.Y"="Target.Y") -> (w752:cluster{"Target.X":dbl, "Target.Y":dbl})  [unwired: 1 in]
        n366 = local write "Image (IMAQ)"(w751) -> ()
        n367 = call "IMAQ Copy"("error in (no error)"=w757, "Image Dst"=w751, "Image Src"=w758) -> ("error out"=w755:errorcluster)  [unwired: 3 in, 1 out]
        n368 = Bundle By Name(cluster=w760, "Image Data.Image Out"=w751, "Image Data.Image Center"=w752) -> (w759:T15)
      }
      frame "Action: IMAQ Histogram Lineprofile" {
        # "Get IMAQ histogram and line profile"
        n369 = Unbundle By Name(w783) -> ("Image Data.Image Out"=w784:T2, "Image Data.valid image"=w780:bool)
        n370 = case shown="True" w780 {
          tunnel: w784 -> [_ w787]
          tunnel: [sgl 0.0 ("Maximal Value") w791] -> w781
          frame False {
          }
          frame True {
            n371 = property on="Image (IMAQ)" class="ImageControl"() -> ("ROI"=w802:T18)  [unwired: 2 in, 2 out]
            n372 = call "GetMaxCounts.vi"("New Image"=w787) -> ("Maximal Value"=w791:sgl, "Color"=w792:u32)
            "Max Counts" <- w791
            n373 = call "IMAQ Histograph"("Image"=w787) -> ("Mean Value"=→"Mean Value" →"Mean Value Graph":sgl, "Histogram Graph"=→"histogram":T6)  [unwired: 7 in, 2 out]
            n374 = call "IMAQ Convert ROI to Line"("ROI Descriptor"=w802) -> ("Line"=w797:T19)  [unwired: 8 in, 1 out]
            n375 = property on="Max Counts" class="Slide (strict)"("Fill Color"=w792) -> ()  [unwired: 2 in, 2 out]
            n376 = Unbundle(w797) -> ("Start X"=w801:i32, "Start Y"=w800:i32, "End X"=w799:i32, "End Y"=w798:i32)
            n377 = Build Array(w801, w800, w799, w798) -> (w796:i32[])
            n378 = call "IMAQ GetImageSize"("Image"=w787) -> ("Y Resolution"=→"Y Resolution":i32, "X Resolution"=→"X Resolution":i32)  [unwired: 3 in, 1 out]
            n379 = call "IMAQ LineProfile"("Line Coordinates"=w796, "Image"=w787) -> ("Line Graph"=→"lineout":cluster{"x0":sgl, "dx":sgl, "Pixels Line":sgl[]})  [unwired: 3 in, 3 out]
            n380 = call "IMAQ Centroid"("Image"=w787) -> ("Centroid"=→"Centroid":cluster{"X Centroid":sgl, "Y Centroid":sgl})  [unwired: 3 in, 1 out]
          }
        }
        n381 = Bundle By Name(cluster=w783, "Image Data.Max count"=w781) -> (w782:T15)
      }
      frame "Action: Lowpass-Sat-Autoscale-Scale" {
        n382 = Unbundle By Name(w805) -> ("IMG Features.Button Label"=w808:string, "Image Data.Image Out"=w807:T2, "Image Data.Max count"=w806:dbl)
        n383 = case shown="\"LowPass\"" w808 {
          tunnel: w807 -> [w813 w823 w832 w838 w846]
          tunnel: w806 -> [w811 _ w831 _ _]
          tunnel: [w812 w822 w832 w837 w846] -> w803
          frame "Autoscale" {
            n384 = Divide(x=256.0, y=w811) -> (x/y=w814:dbl)
            n385 = case shown="True" "Autoscale" {
              tunnel: w813 -> [w817 w818]
              tunnel: w814 -> [_ w821]
              tunnel: [w817 w819] -> w812
              frame False {
              }
              frame True {
                n386 = call "IMAQ Multiply"("Image Src A"=w818, "Constant"=w821, "Image Dst"=w818) -> ("Image Dst Out"=w819:T2, "error out"=w820:errorcluster)  [unwired: 4 in]
                n387 = call <vilib>:"Clear Errors.vi"("error in (no error)"=w820) -> ()  [unwired: 6 in, 1 out]
              }
            }
          }
          frame "Scale" {
            n388 = case shown="True" "Scale" {
              tunnel: w823 -> [w826 w828]
              tunnel: "scale factor" -> [_ w830]
              tunnel: [w826 w827] -> w822
              frame False {
              }
              frame True {
                n389 = call "IMAQ Multiply"("Image Src A"=w828, "Constant"=w830, "Image Dst"=w828) -> ("Image Dst Out"=w827:T2, "error out"=w829:errorcluster)  [unwired: 4 in]
                n390 = call <vilib>:"Clear Errors.vi"("error in (no error)"=w829) -> ()  [unwired: 6 in, 1 out]
              }
            }
          }
          frame "Beep If Sat." {
            n391 = case shown="True" "Beep If Sat." {
              tunnel: w831 -> [_ w836]
              frame False {
              }
              frame True {
                n392 = Greater Or Equal?(x=w836, y="Sat Level") -> (x >= y?=w835:bool)
                n393 = case shown="True" w835 {
                  frame False {
                  }
                  frame True {
                    n394 = call <vilib>:"Beep.vi"() -> ()  [unwired: 12 in]
                  }
                }
              }
            }
          }
          frame "LowPass" {
            n395 = case shown="True" "LowPass" {
              tunnel: w838 -> [_ w843]
              tunnel: [w840 w845] -> w837
              tunnel: w838 -> [w840 w842]
              frame False {
              }
              frame True {
                n396 = call "IMAQ LowPass"("Image Src"=w843, "Size & Tolerance"="Size & Tolerance", "Image Dst"=w842) -> ("Image Dst Out"=w845:T2, "error out"=w841:errorcluster)  [unwired: 4 in]
                n397 = call <vilib>:"Clear Errors.vi"("error in (no error)"=w841) -> ()  [unwired: 6 in, 1 out]
              }
            }
          }
          frame "", Default {
          }
        }
        n398 = local write "Image (IMAQ)"(w803) -> ()
        n399 = Bundle By Name(cluster=w805, "Image Data.Image Out"=w803) -> (w804:T15)
      }
      frame "Action: Analysis" {
        n400 = Multiply(x="SpatialCalibration", y="FWHMx") -> (x*y=→"FWHMx (um)":dbl)
        n401 = Multiply(x="SpatialCalibration", y="FWHMy") -> (x*y=→"FWHMy (um)":dbl)
      }
    }
  }
  n402 = disable-structure shown="Disabled" {
    disable-tunnel: [w855 w865 _] -> _
    frame Disabled {
      w856 = T16 0 items=["Grayscale (U8)", "Grayscale (I16)", "Grayscale (SGL)", "Complex (CSG)", "RGB (U32)", "HSL (U32)", "RGB (U64)", "Grayscale (U16)"] ("Image Type")
      n403 = Create User Event(user event datatype=T20 {"EventEnum"=enum."new data", "Device name"="Device name"} ("New Event")) -> (user event=w863:refnum<user-event>, error out=w862:errorcluster)  [unwired: 1 in]
      "tcp data event" <- w863
      n404 = register-events(w863) -> ()  [unwired: 2 in, 2 out]
      n405 = control-ref of="This Application"() -> (w864:refnum<vi>)
      n406 = control-ref of="This VI"() -> (w859:refnum<vi>)
      n407 = Current VI's Menubar() -> (w860:refnum<k9>)
      n408 = call "GUI_Master_subvi_reentrant_queues.vi"("This Application"=w864, "error in (no error)"=w862, "tcp data event"=w863, "Caller menu reference"=w860, "Caller VI ref"=w859) -> ("error out"=→"error IO 2":errorcluster)  [unwired: 6 in]
      n409 = call "IMAQ Create"("Image Name"="image::1", "Image Type"=w856) -> ("New Image"=w855:T2)  [unwired: 3 in, 1 out]
    }
    frame Disabled {
      n410 = disable-structure shown="Enabled" {
        disable-tunnel: [w866 w873] -> w865
        frame Disabled {
          n411 = call "IMAQ GetFileInfo"("File Path"="File Path") -> ("error out"=w868:errorcluster, "Image Type"=w869:T16)  [unwired: 4 in, 5 out]
          n412 = call "IMAQ Create"("Image Name"="Read Image Source", "Image Type"=w869, "error in (no error)"=w868) -> ("New Image"=w870:T2, "error out"=w871:errorcluster)  [unwired: 2 in]
          n413 = call "IMAQ ReadFile"("File Path"="File Path", "error in (no error)"=w871, "Image"=w870) -> ("Image Out"=w866:T2)  [unwired: 4 in, 4 out]
        }
        frame Enabled {
          n414 = while {
            tunnel: [w880] -> w873
            stop <- w874 stop-if-true
            w876 = 255.0  # A
            w891 = 5.0  # No spot sizes 2
            w890 = 15.0  # w
            w895 = T16 0 items=["Grayscale (U8)", "Grayscale (I16)", "Grayscale (SGL)", "Complex (CSG)", "RGB (U32)", "HSL (U32)", "RGB (U64)", "Grayscale (U16)"] ("Image Type")
            # "This creates an image of a Gaussian beam"
            n415 = Random Number (0-1)() -> (number: 0 to 1=w877:dbl)
            n416 = Multiply(x=w891, y=w890) -> (x*y=w892:dbl)
            n417 = Add(x=0.5, y=w877) -> (x+y=w879:dbl)
            n418 = Random Number (0-1)() -> (number: 0 to 1=w886:dbl)
            n419 = Multiply(x=w876, y=w879) -> (x*y=w875:dbl)
            n420 = Divide(x=w892, y=2.0) -> (x/y=w883:dbl)
            n421 = Initialize Array(0.0 ("element"), w892, w892) -> (w889:dbl[][])
            n422 = Add(x=0.5, y=w886) -> (x+y=w884:dbl)
            n423 = Multiply(x=w883, y=w884) -> (x*y=w882:dbl)
            n424 = for {
              tunnel: w889 -> [w904] mode=indexing
              shift-right: [w902] -> w887
              shift-left: w889 -> [w903]
              tunnel: w875 -> [w901]
              tunnel: w883 -> [w899]
              tunnel: w890 -> [w898]
              tunnel: w882 -> [w897]
              i -> [w900]
              n425 = for {
                tunnel: w904 -> [_] mode=indexing
                shift-right: [w913] -> w902
                shift-left: w903 -> [w914]
                tunnel: w900 -> [w912]
                tunnel: w901 -> [w909]
                tunnel: w900 -> [w908]
                tunnel: w899 -> [w907]
                tunnel: w898 -> [w906]
                tunnel: w897 -> [w905]
                i -> [w911]
                n426 = formula code="I=A*exp((-2/w**2)*((y-x0)**2+(x-y0)**2));"("y"=w911, "A"=w909, "x0"=w907, "x"=w908, "w"=w906, "y0"=w905) -> ("I"=w910:dbl)
                n427 = Replace Array Subset(array=w914, new element=w910, index (row)=w912, index (col)=w911) -> (w913:dbl[][])
              }
            }
            n428 = call "IMAQ Create"("Image Name"="ddfgd", "Image Type"=w895) -> ("New Image"=w894:T2)  [unwired: 3 in, 1 out]
            n429 = call "IMAQ ArrayToImage"("Image Pixels (U8)"=w887, "Image"=w894) -> ("Image Out"=w880:T2)  [unwired: 8 in, 1 out]
            n430 = Wait (ms)(milliseconds to wait=u32 1000) -> ()  [unwired: 1 out]
          }
        }
      }
    }
    frame Enabled {
    }
  }
